vi "Phase_Average_SJ_AM.vi"() -> (5 "Plug in titles":string[](array[string])=["Synthetic_Jet:Frequency:Hz", "Syntehtic_Jet:Num_of:Bins", "Synthetic_Jet:Alanysis:Channels", "Synthetic_Jet:Data:Cluster", "Synethic_Jet:PA_Max_U:U", "Synethic_Jet:PA_Mean_U:U", "Synethic_Jet:PA_Data_Points_Max:U", "Synethic_Jet:PA_Data_Points_Min:U", "Synethic_Jet:PA_Uo:U", "Synethic_Jet:PA_Tb/T:U", "Synethic_Jet:PA_Max_U:V", "Synethic_Jet:PA_Mean_U:V", "Synethic_Jet:PA_Data_Points_Max:V", "Synethic_Jet:PA_Data_Points_Min:V", "Synethic_Jet:PA_Uo:V", "Synethic_Jet:PA_Tb/T:V", "Synethic_Jet:PA_Max_U:Vin", "Synethic_Jet:PA_Mean_U:Vin", "Synethic_Jet:PA_Data_Points_Max:Vin", "Synethic_Jet:PA_Data_Points_Min:Vin", "Synethic_Jet:PA_Max_U:Current", "Synethic_Jet:PA_Mean_U:Current", "Synethic_Jet:PA_Data_Points_Max:Current", "Synethic_Jet:PA_Data_Points_Min:Current", "Synethic_Jet:PA_Max_U:Pressure", "Synethic_Jet:PA_Mean_U:Pressure", "Synethic_Jet:PA_Data_Points_Max:Pressure", "Synethic_Jet:PA_Data_Points_Min:Pressure", "Synethic_Jet:PA_Max_U:Displacement", "Synethic_Jet:PA_Mean_U:Displacement", "Synethic_Jet:PA_Data_Points_Max:Displacement", "Synethic_Jet:PA_Data_Points_Min:Displacement", "Synthetic_Jet:PA_Corr_Coeff:U_cross_V", "Synthetic_Jet:PA_Corr_Coeff_Max:U_cross_V", "Synthetic_Jet:Phase_Lag:U_cross_V", "Synthetic_Jet:PA_Corr_Coeff:U_cross_Vin", "Synthetic_Jet:PA_Corr_Coeff_Max:U_cross_Vin", "Synthetic_Jet:Phase_Lag:U_cross_Vin", "Synthetic_Jet:PA_Corr_Coeff:U_cross_Current", "Synthetic_Jet:PA_Corr_Coeff_Max:U_cross_Current", "Synthetic_Jet:Phase_Lag:U_cross_Current", "Synthetic_Jet:PA_Corr_Coeff:U_cross_Pressure", "Synthetic_Jet:PA_Corr_Coeff_Max:U_cross_Pressure", "Synthetic_Jet:Phase_Lag:U_cross_Pressure", "Synthetic_Jet:PA_Corr_Coeff:U_cross_Displacement", "Synthetic_Jet:PA_Corr_Coeff_Max:U_cross_Displacement", "Synthetic_Jet:Phase_Lag:U_cross_Displacement", "Synthetic_Jet:PA_Corr_Coeff:V_cross_Vin", "Synthetic_Jet:PA_Corr_Coeff_Max:V_cross_Vin", "Synthetic_Jet:Phase_Lag:V_cross_Vin", "Synthetic_Jet:PA_Corr_Coeff:V_cross_Current", "Synthetic_Jet:PA_Corr_Coeff_Max:V_cross_Current", "Synthetic_Jet:Phase_Lag:V_cross_Current", "Synthetic_Jet:PA_Corr_Coeff:V_cross_Pressure", "Synthetic_Jet:PA_Corr_Coeff_Max:V_cross_Pressure", "Synthetic_Jet:Phase_Lag:V_cross_Pressure", "Synthetic_Jet:PA_Corr_Coeff:V_cross_Displacement", "Synthetic_Jet:PA_Corr_Coeff_Max:V_cross_Displacement", "Synthetic_Jet:Phase_Lag:V_cross_Displacement", "Synthetic_Jet:PA_Corr_Coeff:Vin_cross_Current", "Synthetic_Jet:PA_Corr_Coeff_Max:Vin_cross_Current", "Synthetic_Jet:Phase_Lag:Vin_cross_Current", "Synthetic_Jet:PA_Corr_Coeff:Vin_cross_Pressure", "Synthetic_Jet:PA_Corr_Coeff_Max:Vin_cross_Pressure", "Synthetic_Jet:Phase_Lag:Vin_cross_Pressure", "Synthetic_Jet:PA_Corr_Coeff:Vin_cross_Displacement", "Synthetic_Jet:PA_Corr_Coeff_Max:Vin_cross_Displacement", "Synthetic_Jet:Phase_Lag:Vin_cross_Displacement", "Synthetic_Jet:PA_Corr_Coeff:Current_cross_Pressure", "Synthetic_Jet:PA_Corr_Coeff_Max:Current_cross_Pressure", "Synthetic_Jet:Phase_Lag:Current_cross_Pressure", "Synthetic_Jet:PA_Corr_Coeff:Current_cross_Displacement", "Synthetic_Jet:PA_Corr_Coeff_Max:Current_cross_Displacement", "Synthetic_Jet:Phase_Lag:Current_cross_Displacement", "Synthetic_Jet:PA_Corr_Coeff:Pressure_cross_Displacement", "Synthetic_Jet:PA_Corr_Coeff_Max:Pressure_cross_Displacement", "Synthetic_Jet:Phase_Lag:Pressure_cross_Displacement"], 7 "Plug in values":string[](array[string]))   [LabVIEW 2013]
uses:
  Controls/SJ_Data_Cluster.ctl
  Controls/Stats_Menu.ctl
  Controls/Bin_Cluster.ctl
  <vilib>/Analysis/baseanly.llb/Mean (DBL).vi
  <vilib>/Analysis/baseanly.llb/Scale 1D.vi
  <vilib>/Analysis/1siggen.llb/Ramp Pattern by Samples.vi
  Globals/Meas_global.vi
  Globals/Synthetic_jet_global.vi
  <vilib>/Analysis/1siggen.llb/Ramp Pattern by Delta.vi
  <vilib>/Utility/file.llb/Write To Spreadsheet File (DBL).vi
  <vilib>/Analysis/2dsp.llb/1D Cross Correlation (DBL).vi
  <vilib>/Analysis/NI_AALBase.lvlib
  <vilib>/Analysis/NI_AALPro.lvlib
  <vilib>/Analysis/NI_AAL_SigProc.lvlib
panel:
  in  "AM phase Hz":i32=60
  out "Current Frequency":dbl=800.0
  in  "AM Phase averaging?":bool
  in  "Write out PA data?":bool=TRUE
  in  "Tab Control":T1(tab)=enum."Selected Data"
  in  "Overide Channels?":bool
  in  "SJ Data":T2={"Do (mm)"=3.0, "Dc (mm)"=0.039, "Ho (mm)"=0.01, "Hc (mm)"=0.006, "K"=1.251, "beta"=1.039, "Vc (m^3)"=0.0, "Vo (m^3)"=0.0}
  out "Bin Width":dbl=9.693877554482508e-06
  out "Min Num Data Points":i32=548
  in  "Num Bins":i32=20
  in  "Selected Channels":i32[](array[numeric])
  in  "Overide Bins?":bool
  in  "Overide SJ Data":bool
  out "Samples Per Bin":cluster{dbl[], i32[]}[](graph)=[{[0.0, 3.6, 7.2, 10.799999999999999, 14.4, 18.0, 21.599999999999998, 25.200000000000003, 28.8, 32.4, 36.0, 39.6, 43.199999999999996, 46.800000000000004, 50.400000000000006, 54.0, 57.6, 61.2, 64.8, 68.4, 72.0, 75.6, 79.2, 82.8, 86.39999999999999, 90.0, 93.60000000000001, 97.2, 100.80000000000001, 104.39999999999999, 108.0, 111.6, 115.2, 118.80000000000001, 122.4, 126.00000000000001, 129.6, 133.2, 136.8, 140.4, 144.0, 147.60000000000002, 151.2, 154.8, 158.4, 162.0, 165.6, 169.20000000000002, 172.79999999999998, 176.4, 180.0, 183.6, 187.20000000000002, 190.8, 194.4, 198.00000000000003, 201.60000000000002, 205.20000000000002, 208.79999999999998, 212.39999999999998, 216.0, 219.6, 223.2, 226.8, 230.4, 234.0, 237.60000000000002, 241.20000000000002, 244.8, 248.40000000000003, 252.00000000000003, 255.6, 259.2, 262.8, 266.4, 270.0, 273.6, 277.2, 280.8, 284.40000000000003, 288.0, 291.6, 295.20000000000005, 298.8, 302.4, 306.0, 309.6, 313.2, 316.8, 320.4, 324.0, 327.6, 331.2, 334.8, 338.40000000000003, 342.0, 345.59999999999997, 349.2, 352.8, 356.4], [1358, 1345, 1296, 1279, 1181, 1241, 1218, 1082, 1071, 960, 945, 848, 827, 742, 747, 751, 677, 739, 745, 766, 766, 737, 764, 790, 872, 945, 1003, 1066, 1169, 1174, 1250, 1309, 1280, 1388, 1423, 1525, 1537, 1567, 1651, 1571, 1663, 1750, 1677, 1743, 1772, 1705, 1797, 1760, 1746, 1725, 1725, 1747, 1685, 1690, 1563, 1571, 1574, 1487, 1458, 1301, 1305, 1275, 1247, 1196, 1110, 1139, 1029, 969, 995, 960, 948, 839, 925, 938, 862, 860, 943, 895, 990, 971, 984, 1037, 1058, 1109, 1122, 1164, 1278, 1226, 1300, 1339, 1395, 1341, 1435, 1376, 1395, 1372, 1444, 1337, 1357, 1373]}, {[0.0, 3.6, 7.2, 10.799999999999999, 14.4, 18.0, 21.599999999999998, 25.200000000000003, 28.8, 32.4, 36.0, 39.6, 43.199999999999996, 46.800000000000004, 50.400000000000006, 54.0, 57.6, 61.2, 64.8, 68.4, 72.0, 75.6, 79.2, 82.8, 86.39999999999999, 90.0, 93.60000000000001, 97.2, 100.80000000000001, 104.39999999999999, 108.0, 111.6, 115.2, 118.80000000000001, 122.4, 126.00000000000001, 129.6, 133.2, 136.8, 140.4, 144.0, 147.60000000000002, 151.2, 154.8, 158.4, 162.0, 165.6, 169.20000000000002, 172.79999999999998, 176.4, 180.0, 183.6, 187.20000000000002, 190.8, 194.4, 198.00000000000003, 201.60000000000002, 205.20000000000002, 208.79999999999998, 212.39999999999998, 216.0, 219.6, 223.2, 226.8, 230.4, 234.0, 237.60000000000002, 241.20000000000002, 244.8, 248.40000000000003, 252.00000000000003, 255.6, 259.2, 262.8, 266.4, 270.0, 273.6, 277.2, 280.8, 284.40000000000003, 288.0, 291.6, 295.20000000000005, 298.8, 302.4, 306.0, 309.6, 313.2, 316.8, 320.4, 324.0, 327.6, 331.2, 334.8, 338.40000000000003, 342.0, 345.59999999999997, 349.2, 352.8, 356.4], [1147, 1108, 1116, 1075, 1046, 958, 984, 885, 882, 753, 768, 693, 636, 559, 548, 565, 563, 574, 560, 596, 594, 638, 613, 636, 694, 743, 822, 895, 958, 1079, 1079, 1156, 1163, 1207, 1247, 1248, 1289, 1304, 1365, 1443, 1428, 1457, 1436, 1501, 1564, 1476, 1494, 1421, 1495, 1460, 1460, 1447, 1439, 1424, 1392, 1304, 1278, 1228, 1237, 1132, 1047, 985, 968, 932, 908, 819, 819, 753, 702, 627, 641, 648, 609, 630, 643, 665, 682, 724, 722, 764, 788, 784, 821, 842, 888, 918, 937, 1005, 1043, 1079, 1132, 1099, 1179, 1079, 1153, 1158, 1160, 1177, 1142, 1156]}, {[0.0, 3.6, 7.2, 10.799999999999999, 14.4, 18.0, 21.599999999999998, 25.200000000000003, 28.8, 32.4, 36.0, 39.6, 43.199999999999996, 46.800000000000004, 50.400000000000006, 54.0, 57.6, 61.2, 64.8, 68.4, 72.0, 75.6, 79.2, 82.8, 86.39999999999999, 90.0, 93.60000000000001, 97.2, 100.80000000000001, 104.39999999999999, 108.0, 111.6, 115.2, 118.80000000000001, 122.4, 126.00000000000001, 129.6, 133.2, 136.8, 140.4, 144.0, 147.60000000000002, 151.2, 154.8, 158.4, 162.0, 165.6, 169.20000000000002, 172.79999999999998, 176.4, 180.0, 183.6, 187.20000000000002, 190.8, 194.4, 198.00000000000003, 201.60000000000002, 205.20000000000002, 208.79999999999998, 212.39999999999998, 216.0, 219.6, 223.2, 226.8, 230.4, 234.0, 237.60000000000002, 241.20000000000002, 244.8, 248.40000000000003, 252.00000000000003, 255.6, 259.2, 262.8, 266.4, 270.0, 273.6, 277.2, 280.8, 284.40000000000003, 288.0, 291.6, 295.20000000000005, 298.8, 302.4, 306.0, 309.6, 313.2, 316.8, 320.4, 324.0, 327.6, 331.2, 334.8, 338.40000000000003, 342.0, 345.59999999999997, 349.2, 352.8, 356.4], [1604, 1604, 1600, 1600, 1600, 1608, 1600, 1600, 1600, 1604, 1604, 1604, 1596, 1604, 1600, 1600, 1604, 1600, 1600, 1600, 1604, 1600, 1600, 1604, 1596, 1604, 1604, 1600, 1600, 1600, 1596, 1604, 1592, 1596, 1608, 1600, 1600, 1604, 1596, 1604, 1604, 1600, 1596, 1604, 1604, 1600, 1600, 1600, 1600, 1608, 1596, 1600, 1604, 1600, 1604, 1600, 1596, 1604, 1604, 1600, 1596, 1604, 1600, 1600, 1600, 1596, 1596, 1604, 1600, 1604, 1600, 1596, 1604, 1604, 1600, 1604, 1596, 1600, 1608, 1600, 1596, 1600, 1604, 1604, 1600, 1600, 1596, 1608, 1604, 1596, 1600, 1600, 1604, 1608, 1592, 1600, 1604, 1596, 1596, 1600]}, {[0.0, 3.6, 7.2, 10.799999999999999, 14.4, 18.0, 21.599999999999998, 25.200000000000003, 28.8, 32.4, 36.0, 39.6, 43.199999999999996, 46.800000000000004, 50.400000000000006, 54.0, 57.6, 61.2, 64.8, 68.4, 72.0, 75.6, 79.2, 82.8, 86.39999999999999, 90.0, 93.60000000000001, 97.2, 100.80000000000001, 104.39999999999999, 108.0, 111.6, 115.2, 118.80000000000001, 122.4, 126.00000000000001, 129.6, 133.2, 136.8, 140.4, 144.0, 147.60000000000002, 151.2, 154.8, 158.4, 162.0, 165.6, 169.20000000000002, 172.79999999999998, 176.4, 180.0, 183.6, 187.20000000000002, 190.8, 194.4, 198.00000000000003, 201.60000000000002, 205.20000000000002, 208.79999999999998, 212.39999999999998, 216.0, 219.6, 223.2, 226.8, 230.4, 234.0, 237.60000000000002, 241.20000000000002, 244.8, 248.40000000000003, 252.00000000000003, 255.6, 259.2, 262.8, 266.4, 270.0, 273.6, 277.2, 280.8, 284.40000000000003, 288.0, 291.6, 295.20000000000005, 298.8, 302.4, 306.0, 309.6, 313.2, 316.8, 320.4, 324.0, 327.6, 331.2, 334.8, 338.40000000000003, 342.0, 345.59999999999997, 349.2, 352.8, 356.4], [1604, 1604, 1600, 1600, 1600, 1608, 1600, 1600, 1600, 1604, 1604, 1604, 1596, 1604, 1600, 1600, 1604, 1600, 1600, 1600, 1604, 1600, 1600, 1604, 1596, 1604, 1604, 1600, 1600, 1600, 1596, 1604, 1592, 1596, 1608, 1600, 1600, 1604, 1596, 1604, 1604, 1600, 1596, 1604, 1604, 1600, 1600, 1600, 1600, 1608, 1596, 1600, 1604, 1600, 1604, 1600, 1596, 1604, 1604, 1600, 1596, 1604, 1600, 1600, 1600, 1596, 1596, 1604, 1600, 1604, 1600, 1596, 1604, 1604, 1600, 1604, 1596, 1600, 1608, 1600, 1596, 1600, 1604, 1604, 1600, 1600, 1596, 1608, 1604, 1596, 1600, 1600, 1604, 1608, 1592, 1600, 1604, 1596, 1596, 1600]}, {[0.0, 3.6, 7.2, 10.799999999999999, 14.4, 18.0, 21.599999999999998, 25.200000000000003, 28.8, 32.4, 36.0, 39.6, 43.199999999999996, 46.800000000000004, 50.400000000000006, 54.0, 57.6, 61.2, 64.8, 68.4, 72.0, 75.6, 79.2, 82.8, 86.39999999999999, 90.0, 93.60000000000001, 97.2, 100.80000000000001, 104.39999999999999, 108.0, 111.6, 115.2, 118.80000000000001, 122.4, 126.00000000000001, 129.6, 133.2, 136.8, 140.4, 144.0, 147.60000000000002, 151.2, 154.8, 158.4, 162.0, 165.6, 169.20000000000002, 172.79999999999998, 176.4, 180.0, 183.6, 187.20000000000002, 190.8, 194.4, 198.00000000000003, 201.60000000000002, 205.20000000000002, 208.79999999999998, 212.39999999999998, 216.0, 219.6, 223.2, 226.8, 230.4, 234.0, 237.60000000000002, 241.20000000000002, 244.8, 248.40000000000003, 252.00000000000003, 255.6, 259.2, 262.8, 266.4, 270.0, 273.6, 277.2, 280.8, 284.40000000000003, 288.0, 291.6, 295.20000000000005, 298.8, 302.4, 306.0, 309.6, 313.2, 316.8, 320.4, 324.0, 327.6, 331.2, 334.8, 338.40000000000003, 342.0, 345.59999999999997, 349.2, 352.8, 356.4], [1604, 1604, 1600, 1600, 1600, 1608, 1600, 1600, 1600, 1604, 1604, 1604, 1596, 1604, 1600, 1600, 1604, 1600, 1600, 1600, 1604, 1600, 1600, 1604, 1596, 1604, 1604, 1600, 1600, 1600, 1596, 1604, 1592, 1596, 1608, 1600, 1600, 1604, 1596, 1604, 1604, 1600, 1596, 1604, 1604, 1600, 1600, 1600, 1600, 1608, 1596, 1600, 1604, 1600, 1604, 1600, 1596, 1604, 1604, 1600, 1596, 1604, 1600, 1600, 1600, 1596, 1596, 1604, 1600, 1604, 1600, 1596, 1604, 1604, 1600, 1604, 1596, 1600, 1608, 1600, 1596, 1600, 1604, 1604, 1600, 1600, 1596, 1608, 1604, 1596, 1600, 1600, 1604, 1608, 1592, 1600, 1604, 1596, 1596, 1600]}, {[0.0, 3.6, 7.2, 10.799999999999999, 14.4, 18.0, 21.599999999999998, 25.200000000000003, 28.8, 32.4, 36.0, 39.6, 43.199999999999996, 46.800000000000004, 50.400000000000006, 54.0, 57.6, 61.2, 64.8, 68.4, 72.0, 75.6, 79.2, 82.8, 86.39999999999999, 90.0, 93.60000000000001, 97.2, 100.80000000000001, 104.39999999999999, 108.0, 111.6, 115.2, 118.80000000000001, 122.4, 126.00000000000001, 129.6, 133.2, 136.8, 140.4, 144.0, 147.60000000000002, 151.2, 154.8, 158.4, 162.0, 165.6, 169.20000000000002, 172.79999999999998, 176.4, 180.0, 183.6, 187.20000000000002, 190.8, 194.4, 198.00000000000003, 201.60000000000002, 205.20000000000002, 208.79999999999998, 212.39999999999998, 216.0, 219.6, 223.2, 226.8, 230.4, 234.0, 237.60000000000002, 241.20000000000002, 244.8, 248.40000000000003, 252.00000000000003, 255.6, 259.2, 262.8, 266.4, 270.0, 273.6, 277.2, 280.8, 284.40000000000003, 288.0, 291.6, 295.20000000000005, 298.8, 302.4, 306.0, 309.6, 313.2, 316.8, 320.4, 324.0, 327.6, 331.2, 334.8, 338.40000000000003, 342.0, 345.59999999999997, 349.2, 352.8, 356.4], [1604, 1604, 1600, 1600, 1600, 1608, 1600, 1600, 1600, 1604, 1604, 1604, 1596, 1604, 1600, 1600, 1604, 1600, 1600, 1600, 1604, 1600, 1600, 1604, 1596, 1604, 1604, 1600, 1600, 1600, 1596, 1604, 1592, 1596, 1608, 1600, 1600, 1604, 1596, 1604, 1604, 1600, 1596, 1604, 1604, 1600, 1600, 1600, 1600, 1608, 1596, 1600, 1604, 1600, 1604, 1600, 1596, 1604, 1604, 1600, 1596, 1604, 1600, 1600, 1600, 1596, 1596, 1604, 1600, 1604, 1600, 1596, 1604, 1604, 1600, 1604, 1596, 1600, 1608, 1600, 1596, 1600, 1604, 1604, 1600, 1600, 1596, 1608, 1604, 1596, 1600, 1600, 1604, 1608, 1592, 1600, 1604, 1596, 1596, 1600]}]
  out "Engineering Values Scaled":cluster{dbl[], "Y=(X-offset)/scale":dbl[]}[](graph)=[{[0.0, 3.6, 7.2, 10.799999999999999, 14.4, 18.0, 21.599999999999998, 25.200000000000003, 28.8, 32.4, 36.0, 39.6, 43.199999999999996, 46.800000000000004, 50.400000000000006, 54.0, 57.6, 61.2, 64.8, 68.4, 72.0, 75.6, 79.2, 82.8, 86.39999999999999, 90.0, 93.60000000000001, 97.2, 100.80000000000001, 104.39999999999999, 108.0, 111.6, 115.2, 118.80000000000001, 122.4, 126.00000000000001, 129.6, 133.2, 136.8, 140.4, 144.0, 147.60000000000002, 151.2, 154.8, 158.4, 162.0, 165.6, 169.20000000000002, 172.79999999999998, 176.4, 180.0, 183.6, 187.20000000000002, 190.8, 194.4, 198.00000000000003, 201.60000000000002, 205.20000000000002, 208.79999999999998, 212.39999999999998, 216.0, 219.6, 223.2, 226.8, 230.4, 234.0, 237.60000000000002, 241.20000000000002, 244.8, 248.40000000000003, 252.00000000000003, 255.6, 259.2, 262.8, 266.4, 270.0, 273.6, 277.2, 280.8, 284.40000000000003, 288.0, 291.6, 295.20000000000005, 298.8, 302.4, 306.0, 309.6, 313.2, 316.8, 320.4, 324.0, 327.6, 331.2, 334.8, 338.40000000000003, 342.0, 345.59999999999997, 349.2, 352.8, 356.4], "Y=(X-offset)/scale"=[-0.9551153818154593, -0.9386708768164268, -0.9149482127660302, -0.8827086653672397, -0.8571546888473836, -0.8212304216223307, -0.7845060998363727, -0.748651473112596, -0.7025889549208455, -0.6484101862421825, -0.6020642757553747, -0.5570629113828607, -0.48394929325128827, -0.4161715285035951, -0.35985820573777677, -0.2971562326810696, -0.23383278861290493, -0.1878049478017613, -0.14399418919574525, -0.10176114549965982, -0.05340825159098972, 0.0031119310172862944, 0.0898140329754603, 0.16655011360172153, 0.2335979115701082, 0.2849005543486347, 0.3395231481920418, 0.37670823157269784, 0.43078592238789737, 0.4894409536702755, 0.5308781549353541, 0.5685469269508053, 0.6121523593369985, 0.6549610151521917, 0.6906786996134701, 0.7304874396585026, 0.7772210570077172, 0.7921324647883226, 0.8357876373822483, 0.8726159685492605, 0.8971448098950745, 0.9112423741948901, 0.9387797319740145, 0.9692072065965601, 0.9806209311434405, 0.9802782784752133, 0.982207601694826, 1.0, 0.9923989104538731, 0.9934869697759626, 0.99168135356283, 0.9699166080066824, 0.9465766839373022, 0.9361942960185334, 0.8614870493369937, 0.841171792656405, 0.8129017211569531, 0.7586134580175187, 0.7066499984875707, 0.6716334546351881, 0.60763394011458, 0.538615622218619, 0.46465943995624104, 0.43650233431712127, 0.33454310017245303, 0.3037987239608861, 0.21848497259253033, 0.13518581261223045, 0.10287130243872596, 0.035598747439908165, -0.0422264980405214, -0.11750774774481676, -0.1632930691402038, -0.23950339955887318, -0.2858830534794818, -0.36181374962243146, -0.38659174412235037, -0.42025876301264853, -0.49695360086112367, -0.5489646663866689, -0.5999064227716845, -0.66043042114079, -0.7012963181146216, -0.7535927425911034, -0.7947263878889465, -0.8028301348596579, -0.852104364406295, -0.8696631708281138, -0.8996700970639971, -0.935762520845454, -0.9496371590192277, -0.9516459155006031, -0.9763778733099013, -0.9792522871844971, -0.9968488820233004, -1.0, -0.982250992744951, -0.9920432258770852, -0.9810909213509464, -0.9782577963358422]}, {[0.0, 3.6, 7.2, 10.799999999999999, 14.4, 18.0, 21.599999999999998, 25.200000000000003, 28.8, 32.4, 36.0, 39.6, 43.199999999999996, 46.800000000000004, 50.400000000000006, 54.0, 57.6, 61.2, 64.8, 68.4, 72.0, 75.6, 79.2, 82.8, 86.39999999999999, 90.0, 93.60000000000001, 97.2, 100.80000000000001, 104.39999999999999, 108.0, 111.6, 115.2, 118.80000000000001, 122.4, 126.00000000000001, 129.6, 133.2, 136.8, 140.4, 144.0, 147.60000000000002, 151.2, 154.8, 158.4, 162.0, 165.6, 169.20000000000002, 172.79999999999998, 176.4, 180.0, 183.6, 187.20000000000002, 190.8, 194.4, 198.00000000000003, 201.60000000000002, 205.20000000000002, 208.79999999999998, 212.39999999999998, 216.0, 219.6, 223.2, 226.8, 230.4, 234.0, 237.60000000000002, 241.20000000000002, 244.8, 248.40000000000003, 252.00000000000003, 255.6, 259.2, 262.8, 266.4, 270.0, 273.6, 277.2, 280.8, 284.40000000000003, 288.0, 291.6, 295.20000000000005, 298.8, 302.4, 306.0, 309.6, 313.2, 316.8, 320.4, 324.0, 327.6, 331.2, 334.8, 338.40000000000003, 342.0, 345.59999999999997, 349.2, 352.8, 356.4], "Y=(X-offset)/scale"=[-0.6000257655960964, -0.6296084547831131, -0.5644188522659417, -0.5471668426469449, -0.5301005517796318, -0.5217383066292558, -0.4622577642837686, -0.3879637776401403, -0.41150371567583416, -0.3919780554602071, -0.34346035985346257, -0.254251186050764, -0.16933160610108522, -0.16358783981514913, -0.19775129670736702, -0.11171513893076099, -0.07987388867123553, -0.0038315286054692336, -0.04427218846366556, 0.04326943351900303, 0.06364948012281159, 0.04439754383546602, 0.13634659123892143, 0.2018024685577136, 0.28603171816787276, 0.25359032504604373, 0.30261797802126983, 0.37211497845990044, 0.38811857241522246, 0.47416342564524555, 0.48855942251936385, 0.509681101698175, 0.548928600269913, 0.5762077937057899, 0.623049168889291, 0.65962227137938, 0.7496236779793469, 0.6835564674541392, 0.7872377845809949, 0.8752846647101659, 0.9058482192741587, 0.9024524092422583, 0.9954677709139663, 0.8961181525300512, 1.0, 0.9126293702045721, 0.9513759030893776, 0.9082778122911612, 0.8899531986178352, 0.8542600336388043, 0.8869169285396474, 0.7872321008706873, 0.7618678948362775, 0.6769274050542455, 0.5582685539747775, 0.5318027924828322, 0.3768582075706238, 0.3905102299559355, 0.246521072626692, 0.23616866065979547, 0.10754072961511849, 0.07637840202411009, -0.009571846812151478, -0.16938387752406225, -0.08186540292904956, -0.2733266546034608, -0.3631519879569536, -0.3332127098152006, -0.4563965670684298, -0.5602929817749812, -0.432730610080142, -0.5873973221989619, -0.6776048246187775, -0.6842771834265521, -0.6171245381295548, -0.751123919185737, -0.6775780134848866, -0.6411087785539201, -0.8185144122575803, -0.8082595763243787, -0.8601856909719153, -0.9281689486568823, -0.9399487973293656, -0.9558082481365745, -0.9361486165062145, -0.9404541937899846, -1.0, -0.9254977324397713, -0.9007846729344119, -0.9319768254925832, -0.8836209796140401, -0.8008104857946138, -0.9022650900561288, -0.7892983407156048, -0.802189877344158, -0.7374909344930695, -0.7165791211179161, -0.666500904887512, -0.6822185692774972, -0.737008511025971]}, {[0.0, 3.6, 7.2, 10.799999999999999, 14.4, 18.0, 21.599999999999998, 25.200000000000003, 28.8, 32.4, 36.0, 39.6, 43.199999999999996, 46.800000000000004, 50.400000000000006, 54.0, 57.6, 61.2, 64.8, 68.4, 72.0, 75.6, 79.2, 82.8, 86.39999999999999, 90.0, 93.60000000000001, 97.2, 100.80000000000001, 104.39999999999999, 108.0, 111.6, 115.2, 118.80000000000001, 122.4, 126.00000000000001, 129.6, 133.2, 136.8, 140.4, 144.0, 147.60000000000002, 151.2, 154.8, 158.4, 162.0, 165.6, 169.20000000000002, 172.79999999999998, 176.4, 180.0, 183.6, 187.20000000000002, 190.8, 194.4, 198.00000000000003, 201.60000000000002, 205.20000000000002, 208.79999999999998, 212.39999999999998, 216.0, 219.6, 223.2, 226.8, 230.4, 234.0, 237.60000000000002, 241.20000000000002, 244.8, 248.40000000000003, 252.00000000000003, 255.6, 259.2, 262.8, 266.4, 270.0, 273.6, 277.2, 280.8, 284.40000000000003, 288.0, 291.6, 295.20000000000005, 298.8, 302.4, 306.0, 309.6, 313.2, 316.8, 320.4, 324.0, 327.6, 331.2, 334.8, 338.40000000000003, 342.0, 345.59999999999997, 349.2, 352.8, 356.4], "Y=(X-offset)/scale"=[-0.324332635145967, -0.3838198713757219, -0.44081635783682965, -0.49677620053035504, -0.5506176190745422, -0.6016412934008409, -0.6510998236349615, -0.6979186329701068, -0.7408503368561451, -0.7823676502632549, -0.8194289332341465, -0.8538505515393717, -0.8852000566796311, -0.9121357432391195, -0.9365447196039366, -0.9563984945596902, -0.9730569223136102, -0.9855999607686946, -0.9940970958857072, -0.9990580460582431, -1.0, -0.9969372982284642, -0.9900730345704503, -0.9790274583582089, -0.9647344799818981, -0.9460722420888912, -0.9238348078458232, -0.8981293358072846, -0.8685193839184734, -0.8362910192677246, -0.8004211709195546, -0.7610585566664713, -0.7188260754084056, -0.6742369082784718, -0.6265183604012093, -0.5760227440012722, -0.5243522754029674, -0.46856698484684417, -0.4116453200341878, -0.35429697815097067, -0.29438956022332385, -0.23404576059030877, -0.17156181549709187, -0.10965470570481395, -0.046520785865849255, 0.016289322156093303, 0.0782112916621511, 0.14265292590520148, 0.20374035832669787, 0.2652043243472213, 0.32496108551551306, 0.38355755257856, 0.4416600727262193, 0.4970807895566517, 0.5502506998787882, 0.6011085558610448, 0.6503974820545738, 0.6966019309972807, 0.7404334683585393, 0.7809450544956844, 0.8184384115998369, 0.8528818222435408, 0.8838389751352131, 0.9116270989672535, 0.935110787289453, 0.9559393293824295, 0.9720488882455951, 0.9846819898204856, 0.9939115813890408, 0.9989718552474046, 1.0, 0.9974545776418189, 0.9905248186412435, 0.9797572518002684, 0.9653321284070773, 0.9469355392532751, 0.9247748338013451, 0.8990806357040502, 0.8694072459887088, 0.8364925462174618, 0.8007713907470402, 0.7612211647205798, 0.719129817142212, 0.6734979383918018, 0.6256834923978529, 0.5751178905260256, 0.5226125738268346, 0.4681770170126485, 0.41060550382546346, 0.35334796890568226, 0.29262025753632986, 0.23285060362745555, 0.1712713479675681, 0.10787688697628549, 0.04551789324166519, -0.017619594059556206, -0.07995233700932476, -0.14130155409470893, -0.20370375735350435, -0.26591530181050727]}, {[0.0, 3.6, 7.2, 10.799999999999999, 14.4, 18.0, 21.599999999999998, 25.200000000000003, 28.8, 32.4, 36.0, 39.6, 43.199999999999996, 46.800000000000004, 50.400000000000006, 54.0, 57.6, 61.2, 64.8, 68.4, 72.0, 75.6, 79.2, 82.8, 86.39999999999999, 90.0, 93.60000000000001, 97.2, 100.80000000000001, 104.39999999999999, 108.0, 111.6, 115.2, 118.80000000000001, 122.4, 126.00000000000001, 129.6, 133.2, 136.8, 140.4, 144.0, 147.60000000000002, 151.2, 154.8, 158.4, 162.0, 165.6, 169.20000000000002, 172.79999999999998, 176.4, 180.0, 183.6, 187.20000000000002, 190.8, 194.4, 198.00000000000003, 201.60000000000002, 205.20000000000002, 208.79999999999998, 212.39999999999998, 216.0, 219.6, 223.2, 226.8, 230.4, 234.0, 237.60000000000002, 241.20000000000002, 244.8, 248.40000000000003, 252.00000000000003, 255.6, 259.2, 262.8, 266.4, 270.0, 273.6, 277.2, 280.8, 284.40000000000003, 288.0, 291.6, 295.20000000000005, 298.8, 302.4, 306.0, 309.6, 313.2, 316.8, 320.4, 324.0, 327.6, 331.2, 334.8, 338.40000000000003, 342.0, 345.59999999999997, 349.2, 352.8, 356.4], "Y=(X-offset)/scale"=[-0.999477163867277, -1.0, -0.995833837226098, -0.987898747711675, -0.9753734782715575, -0.9591109182029777, -0.938151115815857, -0.9125929181274602, -0.8834560187312184, -0.8489540333199225, -0.8113916998804199, -0.7695338948729418, -0.7240212666116366, -0.6751376300648789, -0.6223626043144008, -0.5680576186970898, -0.5093095314549057, -0.45057763189459554, -0.38870492872574386, -0.325563456299371, -0.2619475442118494, -0.1959196004083376, -0.1315246843879441, -0.06550485068778504, -0.0021499839154213974, 0.06250834085357543, 0.12457836354506895, 0.18593497538706555, 0.2468153361851179, 0.304587456519989, 0.3615037199868826, 0.41776563104806347, 0.47191895369797676, 0.525011810821948, 0.5755782254341417, 0.6254791331531085, 0.6726956683858427, 0.7191932235530573, 0.7624612688694594, 0.8024041654586451, 0.8400249951807948, 0.8739991890717225, 0.9049408992943399, 0.9313591827122311, 0.9536605117952182, 0.9722781758441066, 0.9860929682515216, 0.9955044678806833, 1.0, 0.9993700137544395, 0.994782094536492, 0.9845809980139224, 0.9697232160151795, 0.9504828474978425, 0.9267307827026403, 0.8993530995614197, 0.8669074775421599, 0.8310851243856565, 0.7918109498119879, 0.7488005048544422, 0.703120115856144, 0.6538080238541689, 0.6025128602542822, 0.5484536263860987, 0.49356912784581364, 0.434318748401323, 0.37703129357358267, 0.31744177168835014, 0.25639689829473994, 0.19636228737389466, 0.13565546010338472, 0.07654853738280328, 0.016945513710682387, -0.04101262290395395, -0.09721489387748518, -0.15191465245710603, -0.2062248937225819, -0.25742165674798384, -0.3079563420450002, -0.35705295347058436, -0.40376923853247726, -0.4498426508681331, -0.4943670108445233, -0.5385492834293556, -0.5806889870930813, -0.6226507252858628, -0.6625263962192042, -0.7011898025065944, -0.7389349961378829, -0.7742398969292655, -0.8091261898864373, -0.8399709398002756, -0.8691024946886746, -0.8967180235917159, -0.9214150454408416, -0.9430295872576268, -0.9607977861913224, -0.9758975154254286, -0.9872712381476475, -0.995898000505844]}, {[0.0, 3.6, 7.2, 10.799999999999999, 14.4, 18.0, 21.599999999999998, 25.200000000000003, 28.8, 32.4, 36.0, 39.6, 43.199999999999996, 46.800000000000004, 50.400000000000006, 54.0, 57.6, 61.2, 64.8, 68.4, 72.0, 75.6, 79.2, 82.8, 86.39999999999999, 90.0, 93.60000000000001, 97.2, 100.80000000000001, 104.39999999999999, 108.0, 111.6, 115.2, 118.80000000000001, 122.4, 126.00000000000001, 129.6, 133.2, 136.8, 140.4, 144.0, 147.60000000000002, 151.2, 154.8, 158.4, 162.0, 165.6, 169.20000000000002, 172.79999999999998, 176.4, 180.0, 183.6, 187.20000000000002, 190.8, 194.4, 198.00000000000003, 201.60000000000002, 205.20000000000002, 208.79999999999998, 212.39999999999998, 216.0, 219.6, 223.2, 226.8, 230.4, 234.0, 237.60000000000002, 241.20000000000002, 244.8, 248.40000000000003, 252.00000000000003, 255.6, 259.2, 262.8, 266.4, 270.0, 273.6, 277.2, 280.8, 284.40000000000003, 288.0, 291.6, 295.20000000000005, 298.8, 302.4, 306.0, 309.6, 313.2, 316.8, 320.4, 324.0, 327.6, 331.2, 334.8, 338.40000000000003, 342.0, 345.59999999999997, 349.2, 352.8, 356.4], "Y=(X-offset)/scale"=[0.24798886036906698, 0.30694086077660476, 0.3642095468100585, 0.4212388206223648, 0.4772455735602993, 0.5311088513860781, 0.5843671486103762, 0.6358303072039728, 0.6837980481639937, 0.7310432746524327, 0.7737311958300097, 0.8140957953828596, 0.8510643564392585, 0.882952084279465, 0.9121717576229643, 0.9362761032577382, 0.9566418759813594, 0.9728068048999052, 0.9847297456081049, 0.9932059588740203, 0.9982521215535534, 1.0, 0.9985958788235885, 0.9941830996390469, 0.987120440473217, 0.9769411681055087, 0.9637931320950248, 0.9479205541098594, 0.9286125464455226, 0.9066092471942216, 0.8811045375226862, 0.8515787428062843, 0.8185573409961007, 0.7822134336490338, 0.7416779590856867, 0.6973765058637093, 0.6505950238320156, 0.5985543258925514, 0.5444814356995393, 0.4888205952477875, 0.4298488359060673, 0.3700411729571332, 0.30752228271061893, 0.2453949285457375, 0.18206421313080534, 0.11903705068725319, 0.057139439971723265, -0.007220101030625045, -0.06813067822715113, -0.1295563755840377, -0.18991733891747972, -0.2494230240775392, -0.30955326493446883, -0.3679785421329789, -0.42548046869675754, -0.4820539905587055, -0.5383762168301456, -0.592769088326793, -0.645628167253372, -0.6956777887504435, -0.7430103899338654, -0.7875506147216481, -0.8280771682974074, -0.8650755752817957, -0.8967911032150638, -0.9254198000347772, -0.948212438469826, -0.9669527091292689, -0.9818466144977595, -0.9920200114248434, -0.9977552151391165, -1.0, -0.9981145809461024, -0.9926946393873112, -0.9840652554597449, -0.9717188643000962, -0.9563437929329474, -0.9374004474906461, -0.914585720841493, -0.8887684842397121, -0.8593105672967526, -0.8257209527528148, -0.7887117372658937, -0.7469700250041118, -0.7020904875255574, -0.6529034827799842, -0.6007122397849494, -0.5454247553519498, -0.4861743282108634, -0.4270266091724415, -0.3642359772912829, -0.3024703661156339, -0.23973300672637374, -0.17567688289612113, -0.1134144061952939, -0.05130225676736532, 0.009671750947260563, 0.06933608631330149, 0.12995528015626395, 0.19053569191894756]}, {[0.0, 3.6, 7.2, 10.799999999999999, 14.4, 18.0, 21.599999999999998, 25.200000000000003, 28.8, 32.4, 36.0, 39.6, 43.199999999999996, 46.800000000000004, 50.400000000000006, 54.0, 57.6, 61.2, 64.8, 68.4, 72.0, 75.6, 79.2, 82.8, 86.39999999999999, 90.0, 93.60000000000001, 97.2, 100.80000000000001, 104.39999999999999, 108.0, 111.6, 115.2, 118.80000000000001, 122.4, 126.00000000000001, 129.6, 133.2, 136.8, 140.4, 144.0, 147.60000000000002, 151.2, 154.8, 158.4, 162.0, 165.6, 169.20000000000002, 172.79999999999998, 176.4, 180.0, 183.6, 187.20000000000002, 190.8, 194.4, 198.00000000000003, 201.60000000000002, 205.20000000000002, 208.79999999999998, 212.39999999999998, 216.0, 219.6, 223.2, 226.8, 230.4, 234.0, 237.60000000000002, 241.20000000000002, 244.8, 248.40000000000003, 252.00000000000003, 255.6, 259.2, 262.8, 266.4, 270.0, 273.6, 277.2, 280.8, 284.40000000000003, 288.0, 291.6, 295.20000000000005, 298.8, 302.4, 306.0, 309.6, 313.2, 316.8, 320.4, 324.0, 327.6, 331.2, 334.8, 338.40000000000003, 342.0, 345.59999999999997, 349.2, 352.8, 356.4], "Y=(X-offset)/scale"=[-0.9740279920181284, -0.9846373610513185, -0.993320779441793, -0.9981881422032391, -1.0, -0.9985034423533582, -0.9966436575584205, -0.9948478632283323, -0.9888871672778952, -0.9802074776349564, -0.9708220034750391, -0.9598702874710158, -0.9472496837993849, -0.9318059159059814, -0.9165205641568439, -0.8989799834382035, -0.8787821491656113, -0.8557927595533076, -0.8321828629012147, -0.8071867299816438, -0.778083232433784, -0.7452078131757824, -0.7114712514890126, -0.6727963459650614, -0.6358055098454907, -0.5922837693334781, -0.5472900118366004, -0.49845943357685313, -0.44754200739559946, -0.39850108326512357, -0.34071476098245435, -0.28347567543415353, -0.22251156195994248, -0.16025195206529771, -0.09802186457986746, -0.03155074190368913, 0.032933808330448476, 0.09959109990319813, 0.16678387404418069, 0.23170146358040958, 0.2950335529132527, 0.35845059714725863, 0.4221270154547499, 0.4819989498155311, 0.5381272323377648, 0.5937365353181965, 0.6457901127738864, 0.6974173369464612, 0.7430674916254536, 0.7896290662788872, 0.8300966893376822, 0.8658249474641341, 0.8982686678667795, 0.9279886120282342, 0.9517741984536113, 0.9717513200542929, 0.9852076702205445, 0.9935630444457303, 1.0, 0.9985171650156098, 0.9922135823209215, 0.9835195039994218, 0.9659403209003125, 0.9461292272727337, 0.9200738168538403, 0.8888674276141129, 0.8498067287997931, 0.8117016667430699, 0.7676870036846396, 0.7141748224755682, 0.6604419498718704, 0.6031335003313849, 0.5428168228520944, 0.4771021367227203, 0.4102029794093248, 0.3388377246912229, 0.2678194184920453, 0.1941434987296745, 0.1200453795998981, 0.04349414815145887, -0.029161554569596376, -0.10413288709716835, -0.17498213828263112, -0.24626789528944998, -0.31451590225673404, -0.3824643427235468, -0.44559201683689925, -0.503743365423006, -0.5628367808231299, -0.6163875399650314, -0.6681927885891562, -0.7150617434577229, -0.7594872366097571, -0.8009598502582057, -0.8366271303783458, -0.8694097045479963, -0.8969538126221946, -0.9223926903176659, -0.9404960974508143, -0.961060804521041]}]
  out "Engineering Values":cluster{dbl[], dbl[]}(graph)={[0.0, 3.6, 7.2, 10.799999999999999, 14.4, 18.0, 21.599999999999998, 25.200000000000003, 28.8, 32.4, 36.0, 39.6, 43.199999999999996, 46.800000000000004, 50.400000000000006, 54.0, 57.6, 61.2, 64.8, 68.4, 72.0, 75.6, 79.2, 82.8, 86.39999999999999, 90.0, 93.60000000000001, 97.2, 100.80000000000001, 104.39999999999999, 108.0, 111.6, 115.2, 118.80000000000001, 122.4, 126.00000000000001, 129.6, 133.2, 136.8, 140.4, 144.0, 147.60000000000002, 151.2, 154.8, 158.4, 162.0, 165.6, 169.20000000000002, 172.79999999999998, 176.4, 180.0, 183.6, 187.20000000000002, 190.8, 194.4, 198.00000000000003, 201.60000000000002, 205.20000000000002, 208.79999999999998, 212.39999999999998, 216.0, 219.6, 223.2, 226.8, 230.4, 234.0, 237.60000000000002, 241.20000000000002, 244.8, 248.40000000000003, 252.00000000000003, 255.6, 259.2, 262.8, 266.4, 270.0, 273.6, 277.2, 280.8, 284.40000000000003, 288.0, 291.6, 295.20000000000005, 298.8, 302.4, 306.0, 309.6, 313.2, 316.8, 320.4, 324.0, 327.6, 331.2, 334.8, 338.40000000000003, 342.0, 345.59999999999997, 349.2, 352.8, 356.4], [-3.4129345079198394, -3.3412517080838695, -3.237842880709583, -3.0973083360014426, -2.9859166836535187, -2.829320175768431, -2.669236171546384, -2.5129432316989937, -2.3121533464653394, -2.0759841318383003, -1.8739589188667278, -1.6777946807306292, -1.35908707268056, -1.0636388397283245, -0.8181649477408169, -0.5448424619494378, -0.268810938572507, -0.06817221457678806, 0.12280208595714834, 0.3068990118243837, 0.5176728122974912, 0.7640484214654104, 1.1419892242071963, 1.4764874111731627, 1.7687536655537712, 1.9923856370582802, 2.230489518034254, 2.392582015741923, 2.628310624570555, 2.8839921952249865, 3.0646199857375125, 3.228820917575184, 3.418900186101924, 3.605506247289413, 3.761202245800331, 3.934731454769414, 4.138446710306242, 4.203446627255555, 4.393742716985177, 4.554280105705182, 4.661203118863906, 4.722655432566134, 4.842692788862879, 4.975328375827054, 5.0250816357838035, 5.0235879877456755, 5.03199804874651, 5.10955641407199, 5.076422708891909, 5.081165639043932, 5.073294825930726, 4.978420708450514, 4.876680272642288, 4.831422684466524, 4.50576833302911, 4.417212643554925, 4.293981334569766, 4.0573348255811705, 3.8308223055333523, 3.6781826302092555, 3.3992040662907965, 3.098348171446738, 2.7759677647358965, 2.6532288821968333, 2.2087811245385116, 2.0747641403735777, 1.7028752593793877, 1.3397681295677217, 1.1989068166427646, 0.9056608299305918, 0.566414893717426, 0.23825842112842593, 0.03867685700082338, -0.2935295463634631, -0.4957018494305457, -0.8266893065380204, -0.9346983965154295, -1.0814553938424425, -1.415773800524059, -1.6424938385879915, -1.8645526799124745, -2.1283812147708008, -2.3065186480997393, -2.534482586698385, -2.7137871545514494, -2.749111980203364, -2.963901950097321, -3.0404420713212703, -3.171244457114342, -3.32857397172566, -3.389054534142446, -3.3978108505400577, -3.505619263216504, -3.518149043494506, -3.594853887191462, -3.6085898408852084, -3.531220620320301, -3.573905680624593, -3.5261637842807394, -3.513813985160611]}
  in  "Plot Channel":u16(ring) items=["LDA (U)", "Gen (Vin)"]
  in  "Plot Data":T3
  out "Phase":T4(graph)
  out "fk":dbl[](array[numeric])
  out "phiK":dbl[](array[numeric])
  out "Ak":dbl[](array[numeric])
  out "Amp":T4(graph)
  in  "index":i32
  out "XY Graph":cluster{"Ramp Pattern":dbl[], "X":dbl[]}(graph)
  out "Data Points":i32[][](array[numeric])=[[1358, 1345, 1296, 1279, 1181, 1241, 1218, 1082, 1071, 960, 945, 848, 827, 742, 747, 751, 677, 739, 745, 766, 766, 737, 764, 790, 872, 945, 1003, 1066, 1169, 1174, 1250, 1309, 1280, 1388, 1423, 1525, 1537, 1567, 1651, 1571, 1663, 1750, 1677, 1743, 1772, 1705, 1797, 1760, 1746, 1725, 1725, 1747, 1685, 1690, 1563, 1571, 1574, 1487, 1458, 1301, 1305, 1275, 1247, 1196, 1110, 1139, 1029, 969, 995, 960, 948, 839, 925, 938, 862, 860, 943, 895, 990, 971, 984, 1037, 1058, 1109, 1122, 1164, 1278, 1226, 1300, 1339, 1395, 1341, 1435, 1376, 1395, 1372, 1444, 1337, 1357, 1373], [1147, 1108, 1116, 1075, 1046, 958, 984, 885, 882, 753, 768, 693, 636, 559, 548, 565, 563, 574, 560, 596, 594, 638, 613, 636, 694, 743, 822, 895, 958, 1079, 1079, 1156, 1163, 1207, 1247, 1248, 1289, 1304, 1365, 1443, 1428, 1457, 1436, 1501, 1564, 1476, 1494, 1421, 1495, 1460, 1460, 1447, 1439, 1424, 1392, 1304, 1278, 1228, 1237, 1132, 1047, 985, 968, 932, 908, 819, 819, 753, 702, 627, 641, 648, 609, 630, 643, 665, 682, 724, 722, 764, 788, 784, 821, 842, 888, 918, 937, 1005, 1043, 1079, 1132, 1099, 1179, 1079, 1153, 1158, 1160, 1177, 1142, 1156], [1604, 1604, 1600, 1600, 1600, 1608, 1600, 1600, 1600, 1604, 1604, 1604, 1596, 1604, 1600, 1600, 1604, 1600, 1600, 1600, 1604, 1600, 1600, 1604, 1596, 1604, 1604, 1600, 1600, 1600, 1596, 1604, 1592, 1596, 1608, 1600, 1600, 1604, 1596, 1604, 1604, 1600, 1596, 1604, 1604, 1600, 1600, 1600, 1600, 1608, 1596, 1600, 1604, 1600, 1604, 1600, 1596, 1604, 1604, 1600, 1596, 1604, 1600, 1600, 1600, 1596, 1596, 1604, 1600, 1604, 1600, 1596, 1604, 1604, 1600, 1604, 1596, 1600, 1608, 1600, 1596, 1600, 1604, 1604, 1600, 1600, 1596, 1608, 1604, 1596, 1600, 1600, 1604, 1608, 1592, 1600, 1604, 1596, 1596, 1600], [1604, 1604, 1600, 1600, 1600, 1608, 1600, 1600, 1600, 1604, 1604, 1604, 1596, 1604, 1600, 1600, 1604, 1600, 1600, 1600, 1604, 1600, 1600, 1604, 1596, 1604, 1604, 1600, 1600, 1600, 1596, 1604, 1592, 1596, 1608, 1600, 1600, 1604, 1596, 1604, 1604, 1600, 1596, 1604, 1604, 1600, 1600, 1600, 1600, 1608, 1596, 1600, 1604, 1600, 1604, 1600, 1596, 1604, 1604, 1600, 1596, 1604, 1600, 1600, 1600, 1596, 1596, 1604, 1600, 1604, 1600, 1596, 1604, 1604, 1600, 1604, 1596, 1600, 1608, 1600, 1596, 1600, 1604, 1604, 1600, 1600, 1596, 1608, 1604, 1596, 1600, 1600, 1604, 1608, 1592, 1600, 1604, 1596, 1596, 1600], [1604, 1604, 1600, 1600, 1600, 1608, 1600, 1600, 1600, 1604, 1604, 1604, 1596, 1604, 1600, 1600, 1604, 1600, 1600, 1600, 1604, 1600, 1600, 1604, 1596, 1604, 1604, 1600, 1600, 1600, 1596, 1604, 1592, 1596, 1608, 1600, 1600, 1604, 1596, 1604, 1604, 1600, 1596, 1604, 1604, 1600, 1600, 1600, 1600, 1608, 1596, 1600, 1604, 1600, 1604, 1600, 1596, 1604, 1604, 1600, 1596, 1604, 1600, 1600, 1600, 1596, 1596, 1604, 1600, 1604, 1600, 1596, 1604, 1604, 1600, 1604, 1596, 1600, 1608, 1600, 1596, 1600, 1604, 1604, 1600, 1600, 1596, 1608, 1604, 1596, 1600, 1600, 1604, 1608, 1592, 1600, 1604, 1596, 1596, 1600], [1604, 1604, 1600, 1600, 1600, 1608, 1600, 1600, 1600, 1604, 1604, 1604, 1596, 1604, 1600, 1600, 1604, 1600, 1600, 1600, 1604, 1600, 1600, 1604, 1596, 1604, 1604, 1600, 1600, 1600, 1596, 1604, 1592, 1596, 1608, 1600, 1600, 1604, 1596, 1604, 1604, 1600, 1596, 1604, 1604, 1600, 1600, 1600, 1600, 1608, 1596, 1600, 1604, 1600, 1604, 1600, 1596, 1604, 1604, 1600, 1596, 1604, 1600, 1600, 1600, 1596, 1596, 1604, 1600, 1604, 1600, 1596, 1604, 1604, 1600, 1604, 1596, 1600, 1608, 1600, 1596, 1600, 1604, 1604, 1600, 1600, 1596, 1608, 1604, 1596, 1600, 1600, 1604, 1608, 1592, 1600, 1604, 1596, 1596, 1600]]
  out "U":dbl[][](array[numeric])=[[-3.4129345079198394, -3.3412517080838695, -3.237842880709583, -3.0973083360014426, -2.9859166836535187, -2.829320175768431, -2.669236171546384, -2.5129432316989937, -2.3121533464653394, -2.0759841318383003, -1.8739589188667278, -1.6777946807306292, -1.35908707268056, -1.0636388397283245, -0.8181649477408169, -0.5448424619494378, -0.268810938572507, -0.06817221457678806, 0.12280208595714834, 0.3068990118243837, 0.5176728122974912, 0.7640484214654104, 1.1419892242071963, 1.4764874111731627, 1.7687536655537712, 1.9923856370582802, 2.230489518034254, 2.392582015741923, 2.628310624570555, 2.8839921952249865, 3.0646199857375125, 3.228820917575184, 3.418900186101924, 3.605506247289413, 3.761202245800331, 3.934731454769414, 4.138446710306242, 4.203446627255555, 4.393742716985177, 4.554280105705182, 4.661203118863906, 4.722655432566134, 4.842692788862879, 4.975328375827054, 5.0250816357838035, 5.0235879877456755, 5.03199804874651, 5.10955641407199, 5.076422708891909, 5.081165639043932, 5.073294825930726, 4.978420708450514, 4.876680272642288, 4.831422684466524, 4.50576833302911, 4.417212643554925, 4.293981334569766, 4.0573348255811705, 3.8308223055333523, 3.6781826302092555, 3.3992040662907965, 3.098348171446738, 2.7759677647358965, 2.6532288821968333, 2.2087811245385116, 2.0747641403735777, 1.7028752593793877, 1.3397681295677217, 1.1989068166427646, 0.9056608299305918, 0.566414893717426, 0.23825842112842593, 0.03867685700082338, -0.2935295463634631, -0.4957018494305457, -0.8266893065380204, -0.9346983965154295, -1.0814553938424425, -1.415773800524059, -1.6424938385879915, -1.8645526799124745, -2.1283812147708008, -2.3065186480997393, -2.534482586698385, -2.7137871545514494, -2.749111980203364, -2.963901950097321, -3.0404420713212703, -3.171244457114342, -3.32857397172566, -3.389054534142446, -3.3978108505400577, -3.505619263216504, -3.518149043494506, -3.594853887191462, -3.6085898408852084, -3.531220620320301, -3.573905680624593, -3.5261637842807394, -3.513813985160611], [-0.4200077572758023, -0.44122827096431866, -0.3944658943656522, -0.3820905317351646, -0.3698483905061325, -0.3638499115795391, -0.32118280802234306, -0.26788959486721575, -0.2847754693783302, -0.27076915178956684, -0.23596601346602158, -0.1719737076329121, -0.11105845083008924, -0.10693828209479256, -0.1314447121913005, -0.06972850200284014, -0.046887857505642776, 0.007659514184652489, -0.021349734118240895, 0.04144638883914862, 0.05606558235447396, 0.04225561481117978, 0.10821331077099833, 0.15516669394235932, 0.2155867569402253, 0.19231561270907652, 0.2274845581183134, 0.2773367551175649, 0.28881659329074266, 0.35053904097800165, 0.36086570353378916, 0.37601689142292555, 0.4041702508222837, 0.4237384007649119, 0.45733906624148596, 0.4835740044215842, 0.5481346016230898, 0.5007426915621356, 0.575116281989454, 0.6382748411454698, 0.6601989577764749, 0.6577630455843821, 0.7244856394337288, 0.6532193010850835, 0.727736737694325, 0.6650632723502117, 0.692857274655635, 0.6619417747174531, 0.6487970023530039, 0.6231932686547025, 0.6466189985093068, 0.575112204900599, 0.556917730491972, 0.49598747446508035, 0.41087006821181205, 0.3918854163951234, 0.2807392097637791, 0.2905321980236355, 0.18724463465214355, 0.17981855183513235, 0.08755003783346924, 0.06519640409075843, 0.003541818855763959, -0.11109594662500463, -0.0483164279544499, -0.18565708979530926, -0.2500913845936301, -0.22861507939314826, -0.31697840270432426, -0.3915062888113033, -0.3000021311744795, -0.4109490116601009, -0.4756574473200575, -0.48044372217559744, -0.43227319853806345, -0.5283948081043567, -0.4756382149226868, -0.44947778392975535, -0.5767359467907794, -0.5693798580688151, -0.6066279533891391, -0.6553942991791939, -0.6638443233951395, -0.675220763542928, -0.6611183444056463, -0.6642068588104594, -0.7069207780145301, -0.653478158968213, -0.635750770690451, -0.6581257987398099, -0.6234387598807544, -0.5640364112119536, -0.6368127164654787, -0.5557784184821881, -0.5650258884387831, -0.5186154761289171, -0.5036148310160348, -0.4676922863719135, -0.4789670190451544, -0.5182694199025035], [-0.005962902694880684, -0.006994368922434381, -0.007982647326339253, -0.008952951067038467, -0.009886522844645007, -0.0107712369481883, -0.011628812570022651, -0.012440617315110522, -0.013185022425456439, -0.013904903014172984, -0.014547519214842338, -0.01514436551381067, -0.015687943562685033, -0.016154989146964296, -0.016578223379467974, -0.01692247367002136, -0.017211318920218363, -0.017428806256617017, -0.017576140516193446, -0.017662159852169724, -0.017678492661363964, -0.01762538759811633, -0.017506366164460885, -0.017314843754799858, -0.017067013708882448, -0.016743423820744712, -0.016357842579071597, -0.015912128036733923, -0.015398712599936037, -0.014839895754282932, -0.01421793817979229, -0.013535418536864737, -0.012803137447939308, -0.012029993107670407, -0.011202587538294147, -0.010327029582384444, -0.0094311005277015, -0.008463823396508606, -0.007476842346596942, -0.006482463020748315, -0.005443711142384791, -0.004397392716641737, -0.0033139656957754436, -0.0022405405874115453, -0.0011458434682604316, -5.676101495210684e-05, 0.0010169217502451978, 0.0021342937040094083, 0.0031935061916661396, 0.00425924750324462, 0.005295387100905992, 0.006311408026740565, 0.007318864265531032, 0.008279819948471545, 0.009201748252679946, 0.01008358718446156, 0.010938221993257441, 0.011739374167533326, 0.012499381748239896, 0.0132018237437582, 0.013851931801580524, 0.014449155964147583, 0.014985930905004637, 0.01546775714331108, 0.015874947541419205, 0.016236099598561506, 0.01651542785385255, 0.01673447682048175, 0.016894511352264507, 0.016982252890078032, 0.01700008018642851, 0.016955944379090218, 0.016835787302930668, 0.016649085377386554, 0.016398964031171966, 0.016079980302611447, 0.015695729483424833, 0.015250210423183507, 0.014735695019741306, 0.014164977612851104, 0.013545598266756935, 0.012859825569554301, 0.012129991637925212, 0.011338767422211345, 0.010509699047922347, 0.009632927593870029, 0.008722522868845374, 0.0077786491575999265, 0.006780400200590205, 0.005787595402689878, 0.004734620221388978, 0.0036982570728058563, 0.0026305167211487343, 0.001531302004332368, 0.0004500415508618359, -0.0006447174255391533, -0.001725522709132289, -0.0027892743560575537, -0.003871284031843999, -0.004949987820056926], [-0.0509787667975431, -0.05100587356289877, -0.05078987625575489, -0.050378476591344805, -0.04972909618612768, -0.04888595361760317, -0.04779927959174752, -0.04647419889381447, -0.04496357817406373, -0.043174801224050874, -0.041227358622000464, -0.039057214617736986, -0.03669758402263296, -0.034163181400718404, -0.03142702727876219, -0.028611551433385986, -0.025565720213430797, -0.022520728253937444, -0.019312899372669813, -0.01603929035800743, -0.012741083723239484, -0.009317823799948301, -0.005979229220472847, -0.0025563897705476665, 0.0007282828070610503, 0.004080533977376609, 0.007298593012349358, 0.010479664816927782, 0.013636045089129982, 0.016631276696136364, 0.01958213587008714, 0.02249906973549201, 0.02530668251974238, 0.02805931480746552, 0.030680962107608185, 0.03326810578784354, 0.03571607650248342, 0.038126771247251175, 0.04037003003979453, 0.04244089442292334, 0.044391369801227445, 0.046152783070721855, 0.0477569753332945, 0.049126647712245744, 0.05028287402626065, 0.051248118429350314, 0.05196435495698812, 0.0524523000245258, 0.052685373690786276, 0.05265271166100886, 0.0524148481280048, 0.051885965917114564, 0.05111565494367806, 0.050118126039086455, 0.048886685427354026, 0.047467272371439356, 0.04578510886389001, 0.04392787662471011, 0.04189168255150877, 0.03966177921021683, 0.0372934509550833, 0.03473683479289667, 0.032077405047019635, 0.02927467035433434, 0.026429149300066727, 0.02335727642764006, 0.020387172606101293, 0.01729771668233603, 0.014132807152022663, 0.011020275309636588, 0.007872891991389989, 0.004808456722277857, 0.001718300789951292, -0.0012865749470842645, -0.004200416734951781, -0.007036359830749954, -0.009852108158482828, -0.012506436265210464, -0.015126438539220508, -0.01767188297654468, -0.020093917909107865, -0.0224826227042666, -0.02479101591382858, -0.027081673389240356, -0.029266432605136554, -0.031441965090207614, -0.03350934411728545, -0.03551387252779318, -0.03747079563052326, -0.039301200229136295, -0.04110990184352959, -0.04270906713842654, -0.04421941076883518, -0.04565115508659845, -0.04693158758609212, -0.048052206985991816, -0.048973410340435064, -0.04975626521917376, -0.050345942966665995, -0.05079320284100726], [233.31913863944476, 295.7666196138201, 356.43097632400065, 416.841725183357, 476.1693241511608, 533.2263534968985, 589.6425307198978, 644.1571289513087, 694.9690534030133, 745.015622847154, 790.2346676148278, 832.9926324877648, 872.1531952720655, 905.9316635827481, 936.883878648928, 962.4174594438359, 983.9907936122244, 1001.1142005214825, 1013.7440961634751, 1022.7228952372775, 1028.068263430813, 1029.9197800082902, 1028.4324033316122, 1023.7579742661732, 1016.2765441054033, 1005.4937053022918, 991.5660739591812, 974.7523525436112, 954.2995022088226, 930.9915465521827, 903.9745689948525, 872.6980814955399, 837.718719522524, 799.2198484596139, 756.2808767693805, 709.3526277177523, 659.7972998419957, 604.6709178362653, 547.3918474363768, 488.4306713761988, 425.9622598878816, 362.6083809981693, 296.3825161891939, 230.57140307379154, 163.48557700126563, 96.72130267039263, 31.15355533703645, -37.022099169672785, -101.54428814244818, -166.6121406413338, -230.55212712698537, -293.58612285590465, -357.281706482234, -419.1712328944718, -480.08265982244353, -540.0106335248538, -599.6724113984762, -657.2904359684147, -713.2837237749551, -766.300971105097, -816.4400960107125, -863.6212742710151, -906.5507960155502, -945.7429744025004, -979.3390324414705, -1009.6652298157944, -1033.8093274747184, -1053.6607775929501, -1069.4377972988673, -1080.2144122849063, -1086.289677286184, -1088.667563683974, -1086.6703512114022, -1080.9290414163988, -1071.7879896299971, -1058.7095356044442, -1042.4228198010408, -1022.3562538504158, -998.1887582860686, -970.8407229292478, -939.6361379258018, -904.0548717996577, -864.8512440343724, -820.6345123834446, -773.0939023370306, -720.9904194729793, -665.7045660425551, -607.1388836503871, -544.375281125654, -481.7204766441207, -415.20675764118937, -349.77883658511564, -283.32154879573585, -215.46730217935706, -149.51305461670353, -83.71804778293743, -19.12866726373699, 44.07338562441554, 108.2869140546797, 172.45936087272344], [-0.04834149322919361, -0.048826267502530954, -0.04922303924523851, -0.04944544382352849, -0.04952823310572497, -0.04945985084440588, -0.04937487163219172, -0.04929281633854434, -0.04902045404829708, -0.04862385268338215, -0.0481950018816458, -0.04769458473609845, -0.047117911047507385, -0.04641223841658145, -0.04571380430012148, -0.04491232192683493, -0.04398942157320853, -0.042938966583009865, -0.04186015874276201, -0.040718009559863315, -0.03938818242017179, -0.03788600472877459, -0.03634447882601438, -0.03457730500416773, -0.032887081424998486, -0.030898441001134976, -0.028842539653276277, -0.026611322319007175, -0.024284750569074993, -0.022043921893517546, -0.019403489431814813, -0.016788061877512042, -0.014002426490840046, -0.011157595940547839, -0.008314114358740878, -0.005276847006417193, -0.0023303521787374844, 0.000715421795541856, 0.003785663593693458, 0.006751945301473301, 0.009645780692552492, 0.012543497930926168, 0.015453066757985566, 0.01818879716591558, 0.020753468758379526, 0.023294426600339837, 0.0256729125505174, 0.028031917125095663, 0.030117811252542367, 0.03224535092501938, 0.03409443945239982, 0.03572697201080891, 0.03720942407118591, 0.03856741852772935, 0.03965425416698299, 0.040567069488709084, 0.041181930971348646, 0.041563713380444296, 0.04185783741756318, 0.04179008218633424, 0.04150205235999115, 0.04110479353267937, 0.04030154729946087, 0.039396318299764185, 0.03820576751273708, 0.036779852868817624, 0.03499505098055045, 0.03325391503634546, 0.031242751485187226, 0.02879761750227364, 0.02634239945968345, 0.023723802454039895, 0.02096775038311346, 0.017965046912596094, 0.014908221358500841, 0.0116473262582104, 0.008402284288829142, 0.005035807889193075, 0.0016500399189746974, -0.0018478181989211126, -0.005167677785313819, -0.008593345526108609, -0.011830662858787037, -0.015087925467352601, -0.018206384056245643, -0.02131115454246944, -0.02419564958171643, -0.026852761203173564, -0.029552918716782405, -0.031999815442541116, -0.03436695449466149, -0.036508539302147314, -0.03853847492725914, -0.04043348452509024, -0.04206323081330674, -0.04356116613080804, -0.04481974003229292, -0.04598211956784874, -0.04680931918833959, -0.04774898307364484]]
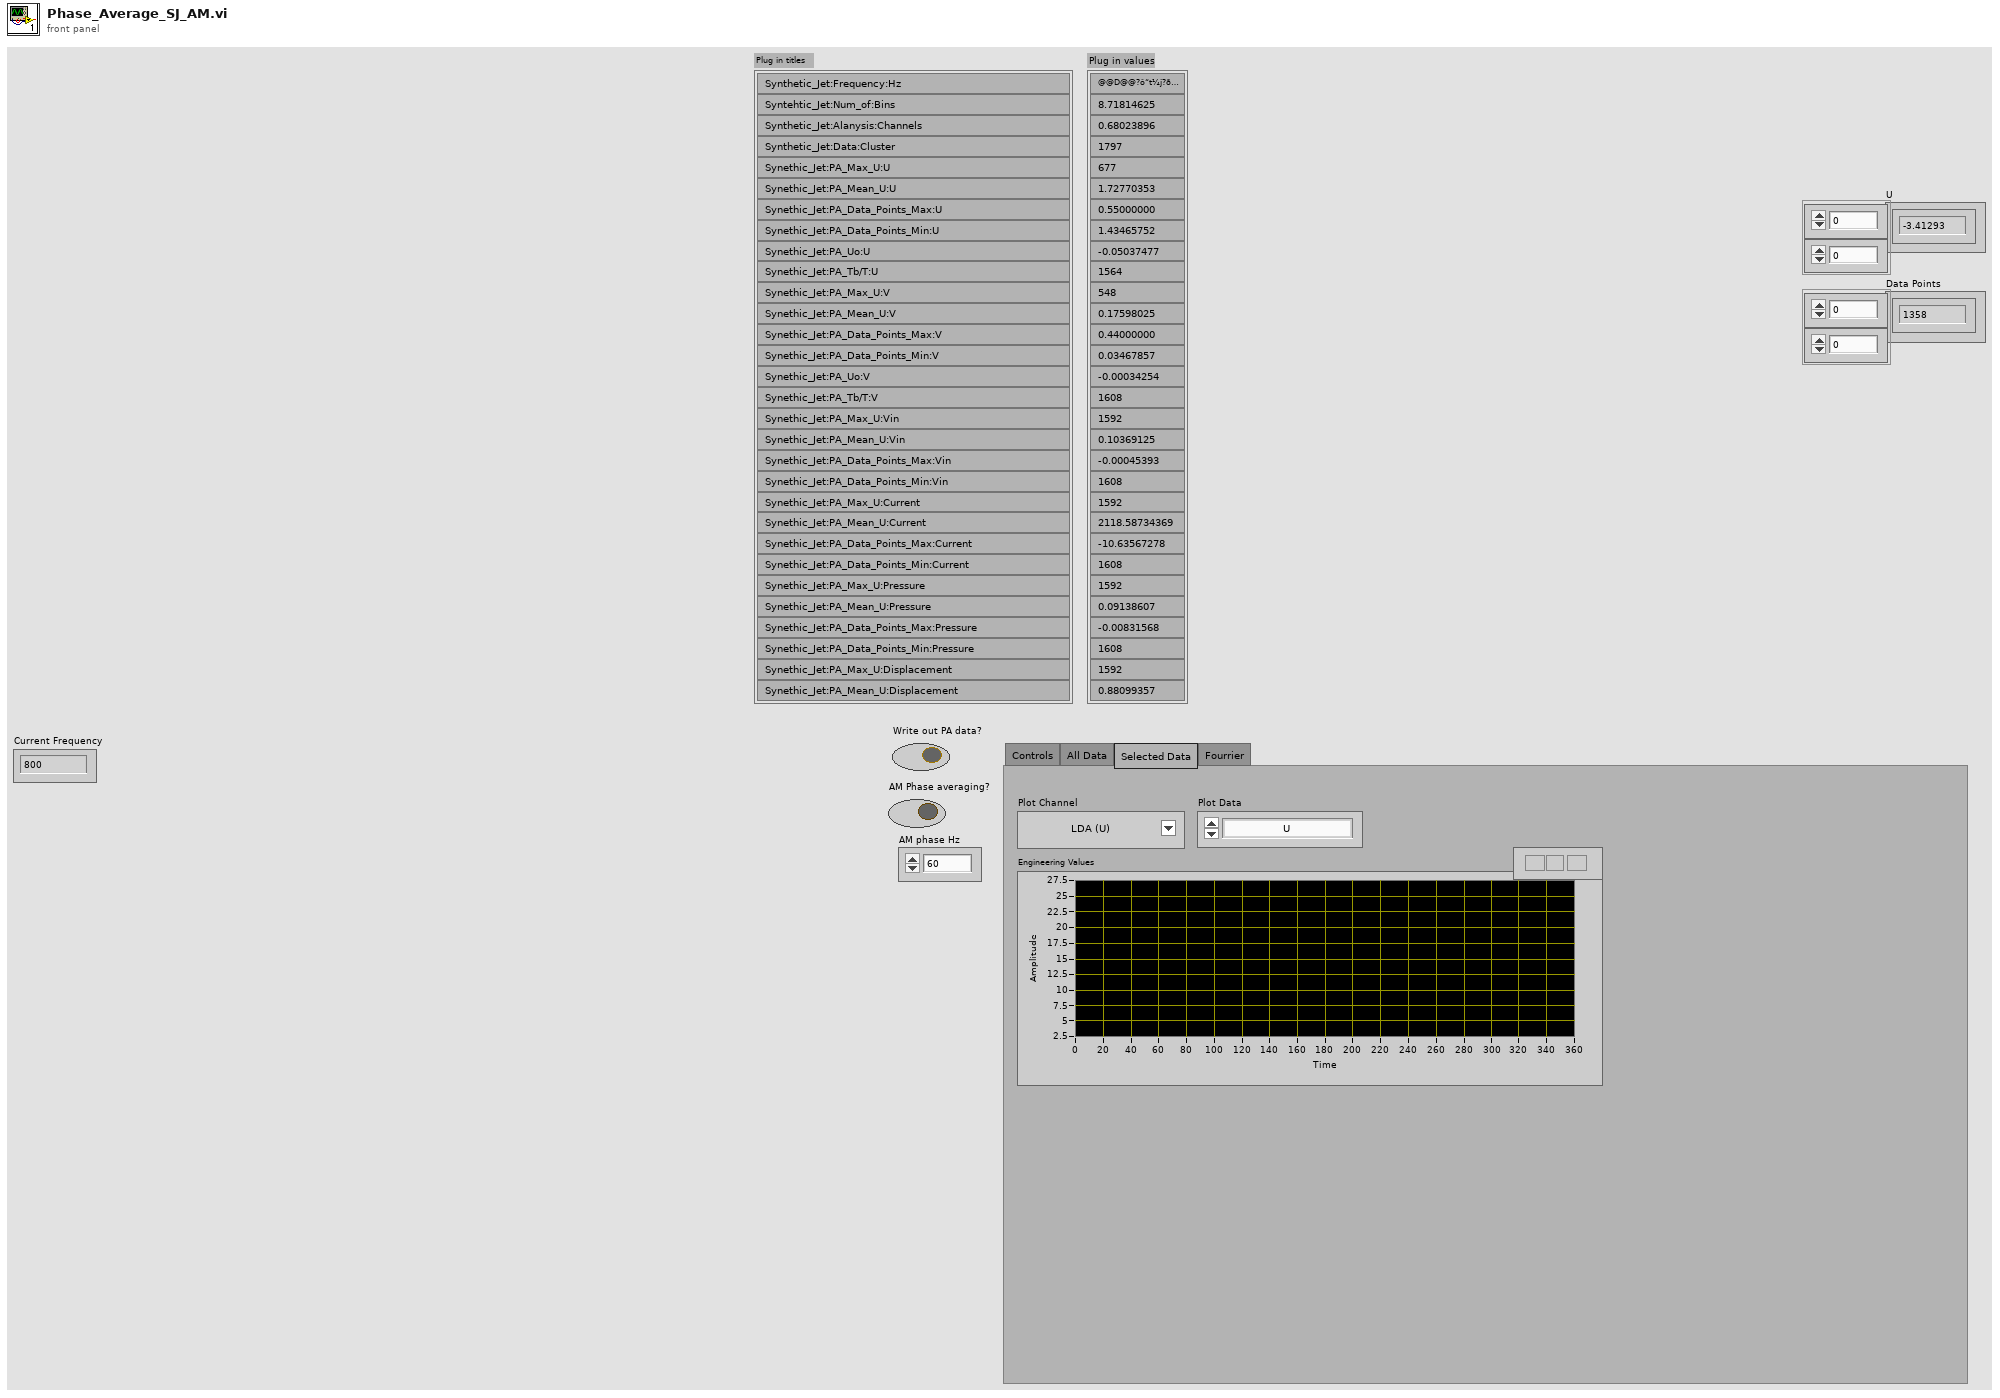
[diagram p1: front panel]
types:
  T1 = enum32{"Controls", "All Data", "Selected Data", "Fourrier"}
  T2 = typedef "SJ_Data_Cluster.ctl" = cluster{"Do (mm)":dbl, "Dc (mm)":dbl, "Ho (mm)":dbl, "Hc (mm)":dbl, "K":dbl, "beta":dbl, "Vc (m^3)":dbl, "Vo (m^3)":dbl}
  T3 = typedef "Stats_Menu.ctl" = enum16{"U", "u^2", "u^3", "u^4", "Skew_u", "Kurt_u", "% u'/U"}
  T4 = cluster{"Ramp Pattern":dbl[], "Amp Spectrum Mag (Vrms)":dbl[]}
  T5 = typedef "Analysis_info_cluster.ctl" = cluster{"Colour":u32, "Inst type":T6, "Inst name":string, "Symbol":string, "Code name":string, "Extra Info":string, "Inst Array":T7, "Extra Titles":string[], "Extra Values":string[], "U":dbl, "u^2":dbl, "u^3":dbl, "u^4":dbl, "Skew_u":dbl, "Kurt_u":dbl, "Sd Error in Mean":dbl, "% u'/U":dbl, "X":dbl, "Y":dbl, "Z":dbl, "Timescale integral to 25%":dbl, "Sd Error in Variance":dbl, "Calib File":path, "Calib Constants":dbl[], "Output Position":bool, "Full Stats":bool, "Av Sampling Rate":dbl, "Av No of Samples":dbl, "Total Meas Time (s)":dbl, "ADAM Ch Name":string}
  T6 = typedef "Inst_type.ctl" = enum16{"Propeller anemometer", "Raw voltage", "Pressure Transducer", "Pitot-static tube", "Preston tube", "Hot wire", "Cross wire 1", "Cross wire 2", "Generic Linear", "Generic Polynomial", "Generic BackPoly", "Fast FID", "Thermocouple", "Cold wire", "Pulsed Wire", "LDA Vel", "LDA Tran time", "LDA Arr time"}
  T7 = typedef "Instrument_Array.ctl" = enum16{"PWA", "LDA", "Analogue"}
  T8 = typedef "Time_Trace_Cluster.ctl" = cluster{"Weighting":dbl[], "Time (s)":dbl[], "Voltage":dbl[], "Eng Values":dbl[]}
  T9 = typedef "Post_Process.ctl" = enum16{"Take New Data", "Post Process Raw Data File"}
  T10 = enum16{"SJ Data Cluster to String", "String to SJ Data Cluster"}
  T11 = typedef "Bin_Cluster.ctl" = cluster{"Start Time":dbl, "End Time":dbl, "Bin Number":i32, "Data Points":i32, "Shift":dbl[], "Stats":cluster{"U":dbl, "u^2":dbl, "u^3":dbl, "u^4":dbl, "Skew_u":dbl, "Kurt_u":dbl, "% u'/U":dbl}, "Channel Name":string, "Bin Centre":dbl, "Symbol":string}
  T12 = cluster{"Ramp Pattern":dbl[], "Amp Spectrum Phase (radians)":dbl[]}
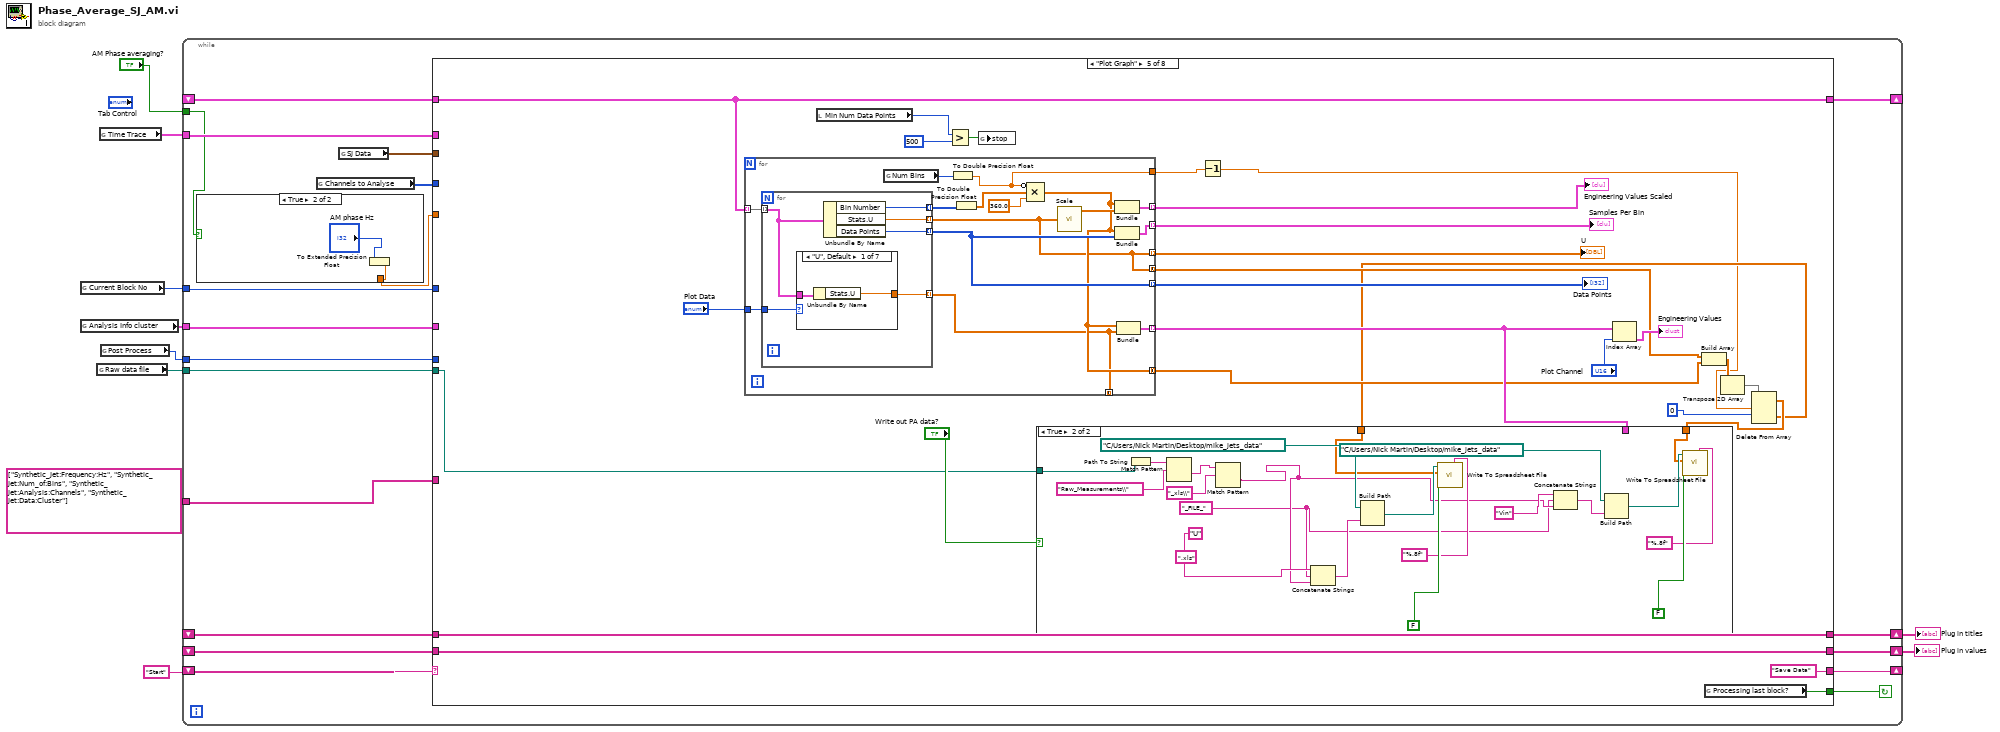
[diagram p0: block diagram]
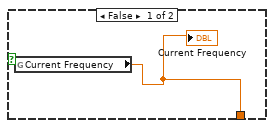
[diagram p2: hidden frame]
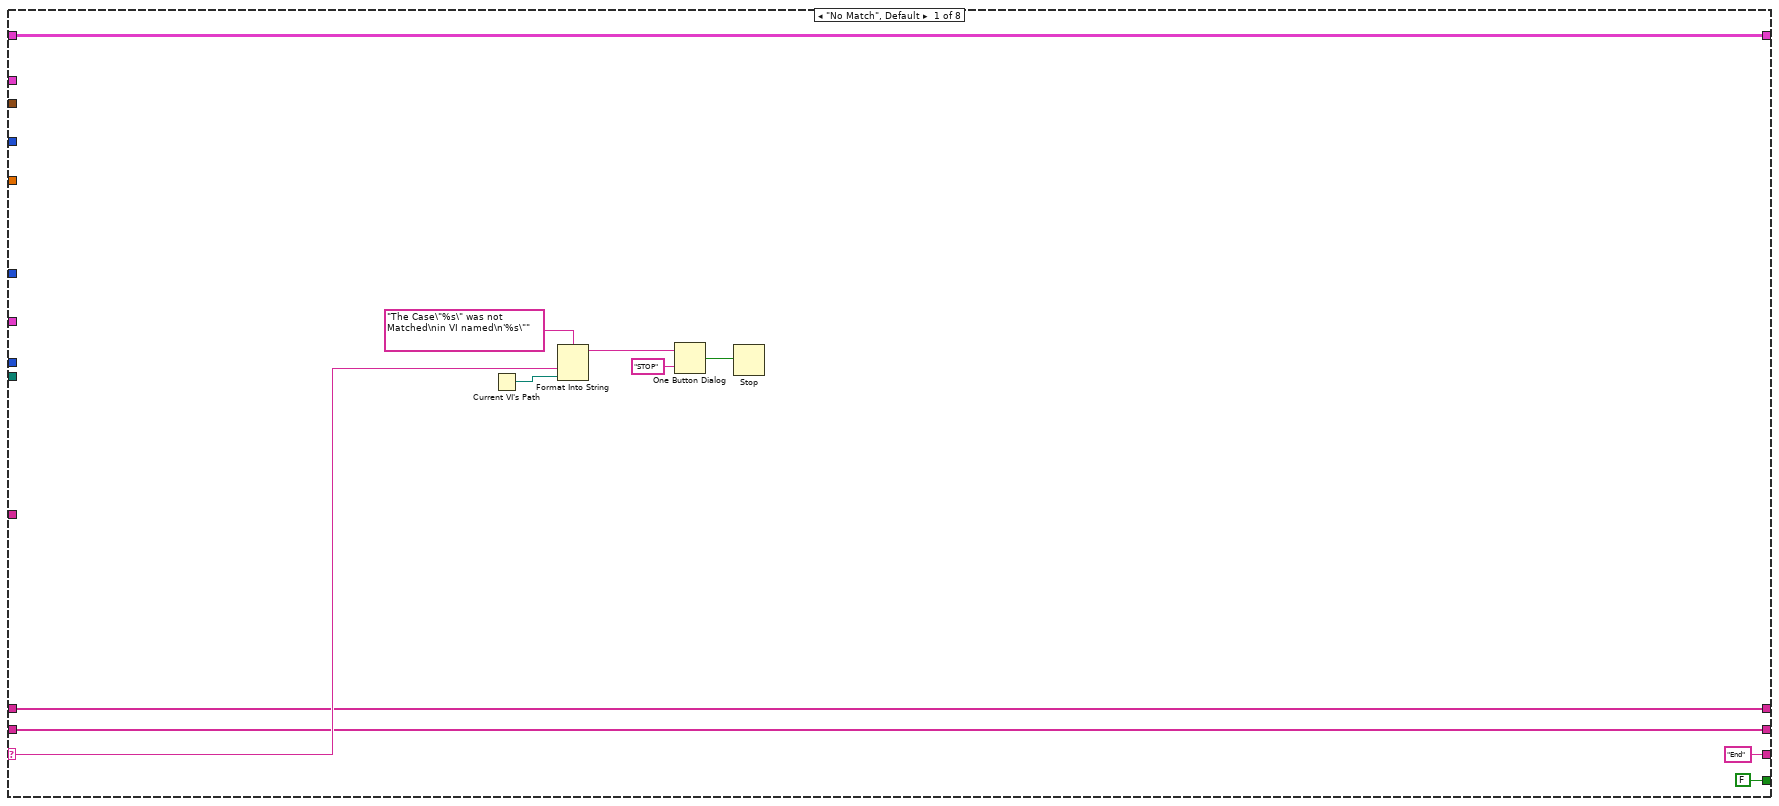
[diagram p3: hidden frame]
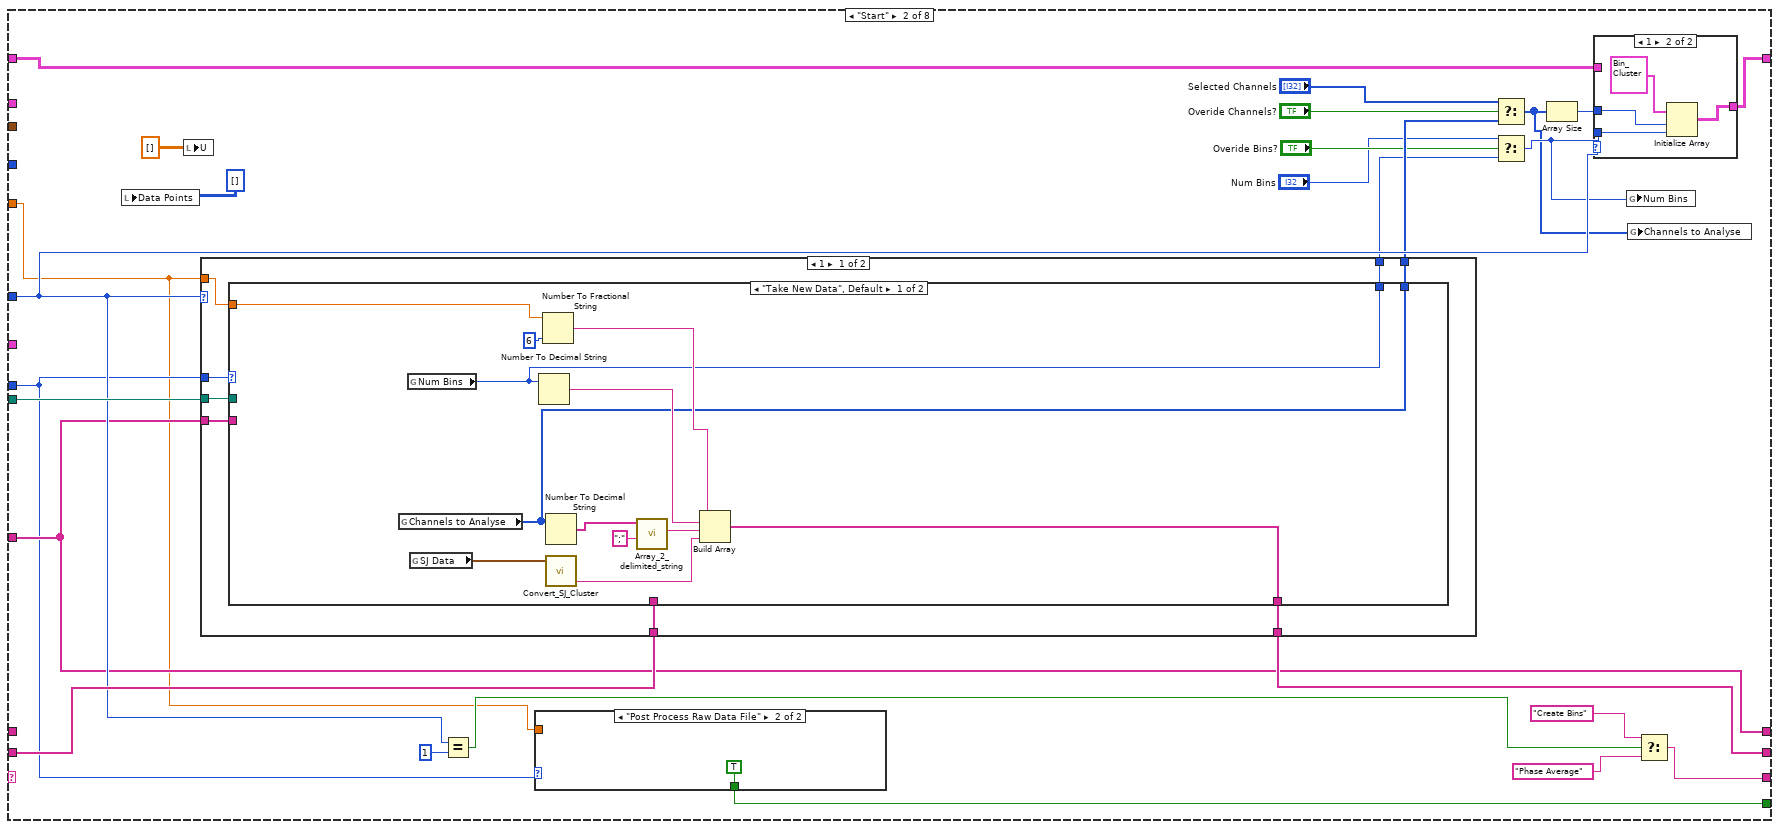
[diagram p4: hidden frame]
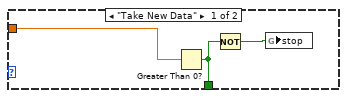
[diagram p5: hidden frame]
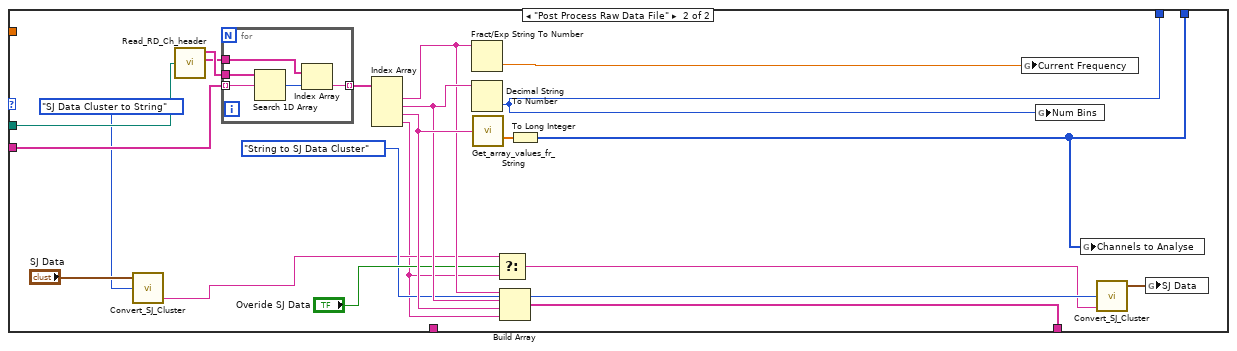
[diagram p6: hidden frame]
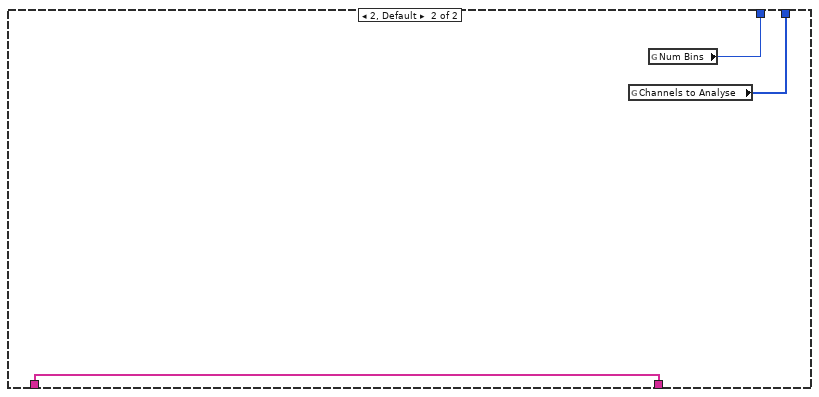
[diagram p7: hidden frame]
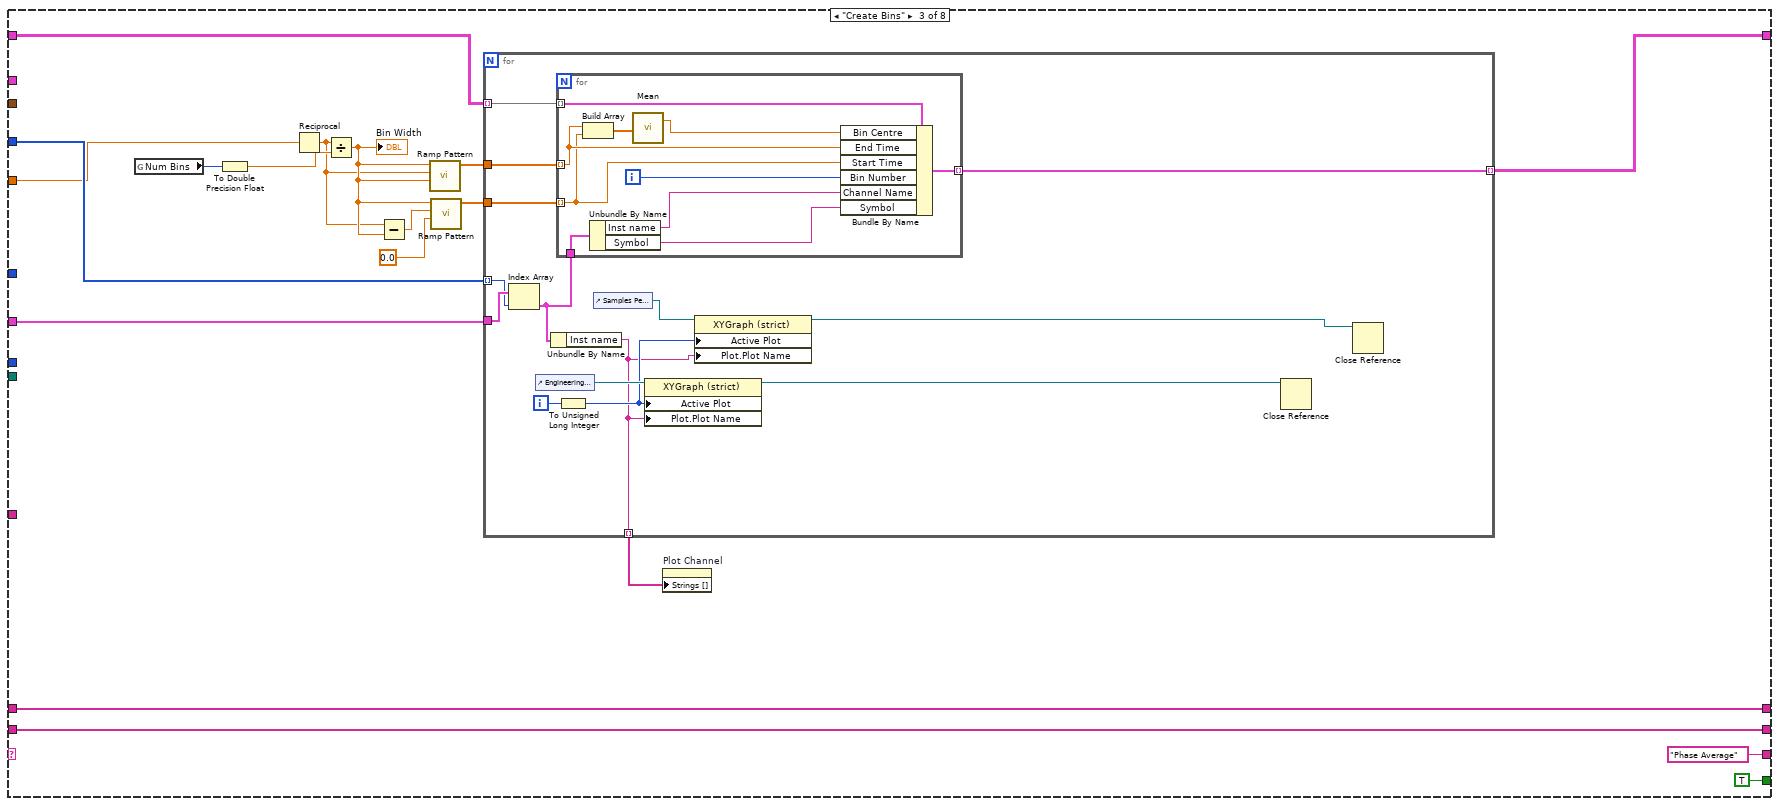
[diagram p9: hidden frame]
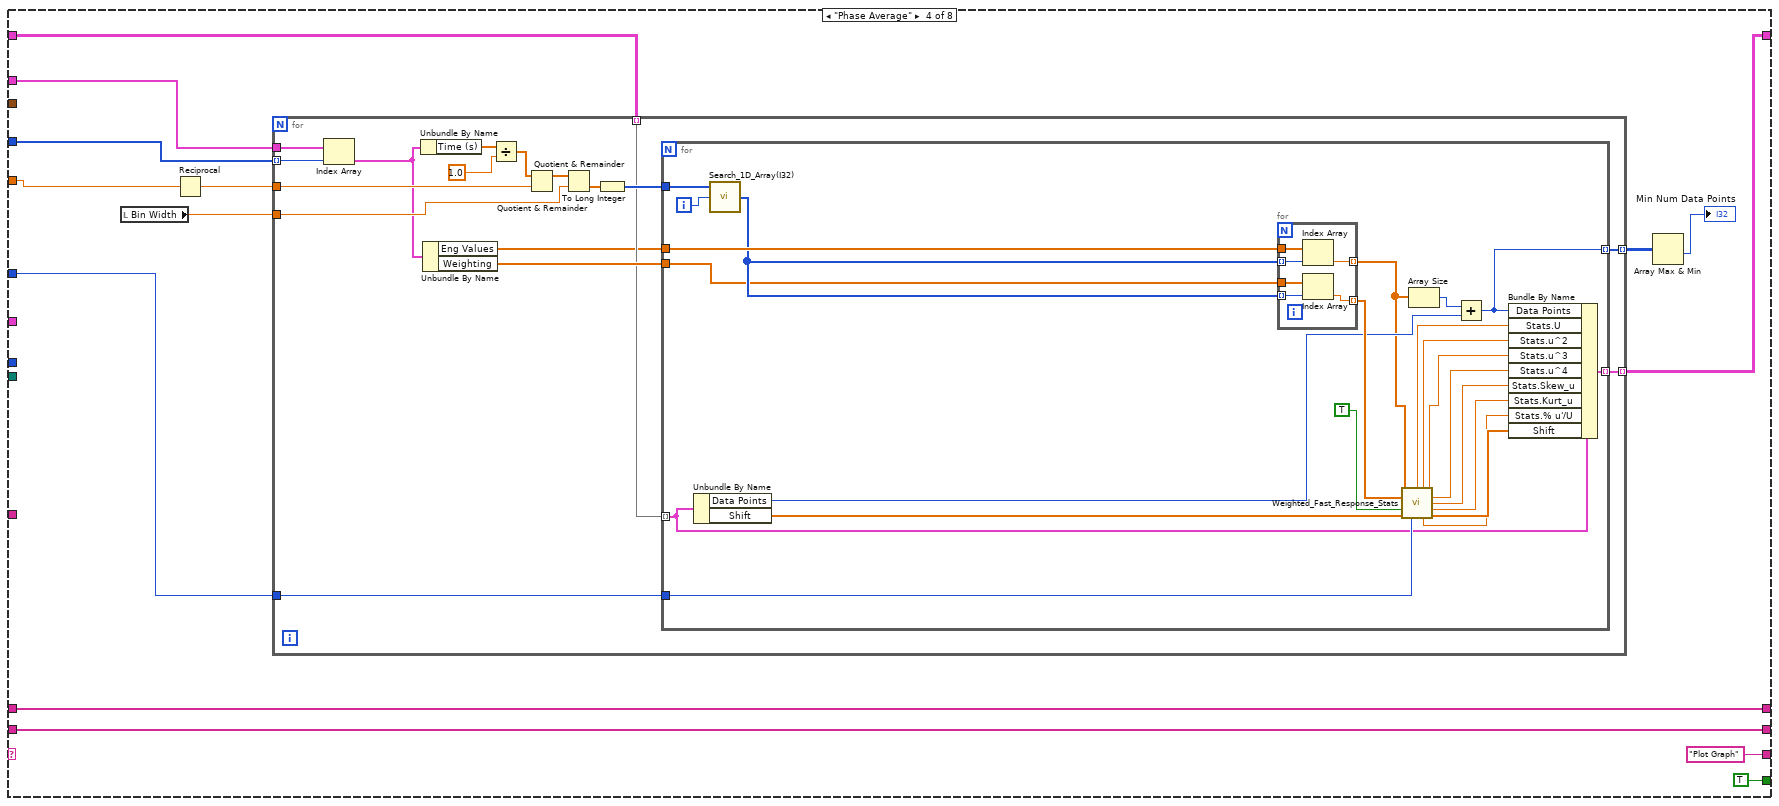
[diagram p10: hidden frame]
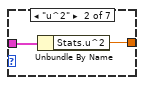
[diagram p12: hidden frame]
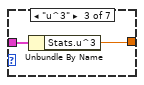
[diagram p13: hidden frame]
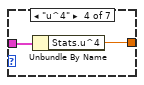
[diagram p14: hidden frame]
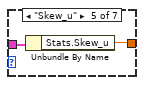
[diagram p15: hidden frame]
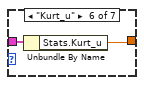
[diagram p16: hidden frame]
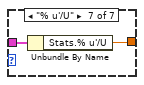
[diagram p17: hidden frame]
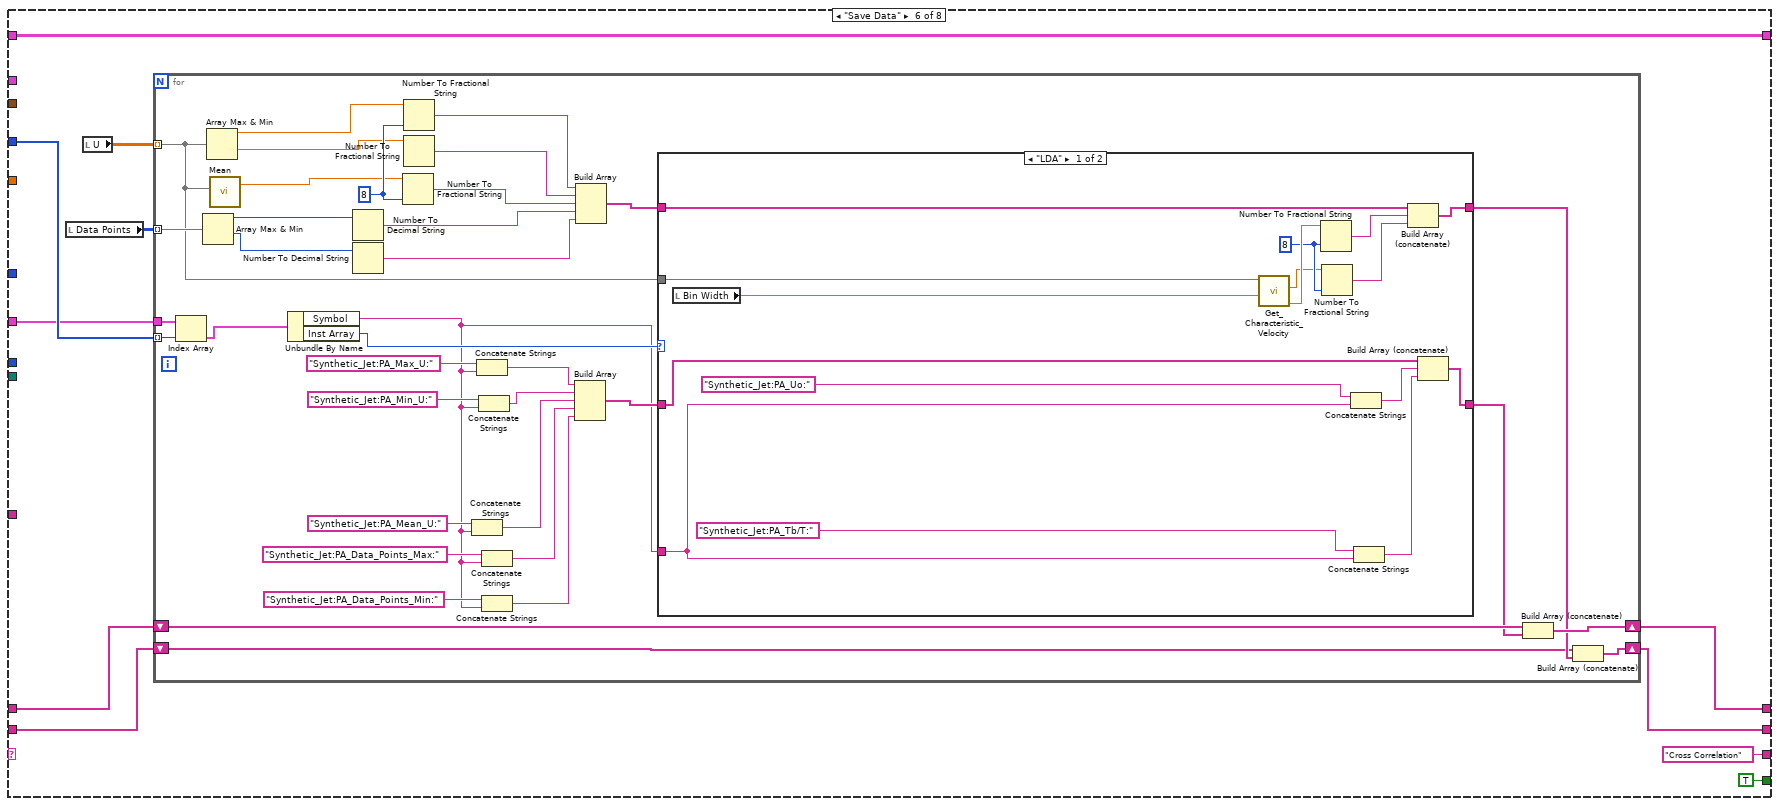
[diagram p18: hidden frame]
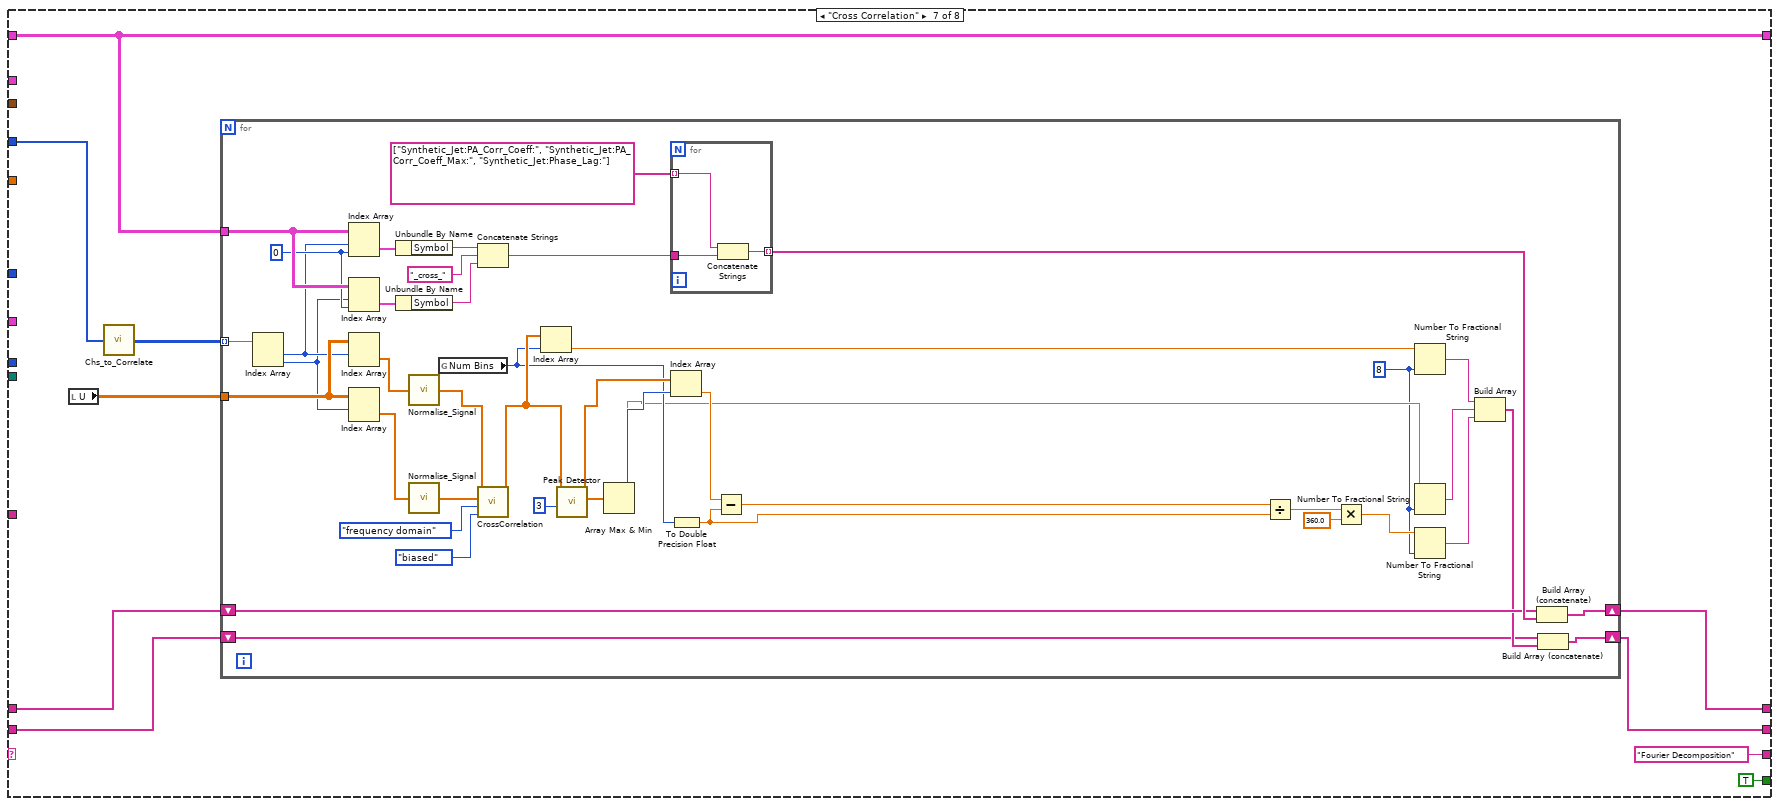
[diagram p20: hidden frame]
diagram:
  n1 = global read "Meas_global.vi" "Current Block No"() -> (w8:i32)
  n2 = global read "Meas_global.vi" "Analysis Info cluster"() -> (w7:T5[])
  n3 = global read "Meas_global.vi" "Raw data file"() -> (w5:path)
  n4 = global read "Meas_global.vi" "Time Trace"() -> (w9:T8[])
  n5 = global read "Meas_global.vi" "Post Process"() -> (w6:T9)
  n6 = while {
    shift-right: [w27] -> _
    shift-left: "Start" -> [w28]
    tunnel: w9 -> [w26]
    shift-right: [w23] -> _
    shift-left: _ -> [w25]
    tunnel: w8 -> [w24]
    tunnel: w7 -> [w22]
    tunnel: w6 -> [w21]
    tunnel: w5 -> [w20]
    shift-right: [w18] -> w4
    shift-left: _ -> [w19]
    shift-right: [w16] -> w3
    shift-left: _ -> [w17]
    tunnel: string[] ["Synthetic_Jet:Frequency:Hz", "Synthetic_Jet:Num_of:Bins", "Synthetic_Jet:Analysis:Channels", "Synthetic_Jet:Data:Cluster"] ("Desired Ch Names") -> [w13]
    tunnel: "AM Phase averaging?" -> [w11]
    stop <- w29 continue-if-true
    n7 = case shown="True" w11 {
      tunnel: [w30 w31] -> w12
      frame False {
        n8 = global read "Synthetic_jet_global.vi" "Current Frequency"() -> (w30:dbl)
        "Current Frequency" <- w30
      }
      frame True {
        n9 = To Extended Precision Float(1:"AM phase Hz") -> (0:w31:ext)
      }
    }
    n10 = global read "Synthetic_jet_global.vi" "Channels to Analyse"() -> (w15:i32[])
    n11 = global read "Synthetic_jet_global.vi" "SJ Data"() -> (w14:T2)
    n12 = case shown="\"Plot Graph\"" w28 {
      selector: w28 -> [w38 _ _ _ _ _ _ _]
      tunnel: [FALSE w46 TRUE TRUE w248 TRUE ("Processing last block?") TRUE ("Processing last block?") FALSE ("Processing last block?")] -> w29
      tunnel: ["End" w62 "Phase Average" "Plot Graph" "Save Data" "Cross Correlation" "Fourier Decomposition" "End"] -> w27
      tunnel: w26 -> [_ _ _ w172 _ _ _ _]
      tunnel: w25 -> [w35 w68 w137 w178 w255 w321 w384 w447]
      tunnel: [w35 w69 w136 w177 w255 w321 w384 w447] -> w23
      tunnel: w24 -> [_ w60 _ w179 _ _ _ _]
      tunnel: w22 -> [_ _ w135 _ _ w313 _ w437]
      tunnel: w21 -> [_ w45 _ _ _ _ _ _]
      tunnel: w20 -> [_ w66 _ _ w230 _ _ _]
      tunnel: [w34 w55 w132 w175 w253 w318 w382 w448] -> w18
      tunnel: w19 -> [w34 _ w132 w175 w253 w319 w383 w449]
      tunnel: [w33 w64 w131 w174 w252 w316 w380 w439] -> w16
      tunnel: w17 -> [w33 w65 w131 w174 w252 w317 w379 w438]
      tunnel: w15 -> [_ _ w130 w171 _ w314 w386 w436]
      tunnel: w14 -> [_ _ _ _ _ _ _ _]
      tunnel: w13 -> [_ w55 _ _ _ _ _ _]
      tunnel: w12 -> [_ w44 w128 w170 _ _ _ w434]
      frame "No Match", Default {
        n13 = Current VI's Path() -> (path=w43:path)
        n14 = Format Into String(format string="The Case\"%s\" was not Matched\nin VI named\n'%s\"" ("Format String"), w38, w43) -> (resulting string=w40:string)  [unwired: 2 in, 1 out]
        n15 = One Button Dialog(message=w40, button name ("OK")="STOP") -> (true=w42:bool)
        n16 = Stop(stop? (T)=w42) -> ()
      }
      frame "Start" {
        n17 = local write "Data Points"(i32[][] [] ("Data Points")) -> ()
        n18 = local write "U"(dbl[][] [] ("U")) -> ()
        n19 = case shown="1" w60 {
          tunnel: w45 -> [w81 _]
          tunnel: [w80 w121] -> w51
          tunnel: [w79 w122] -> w64
          tunnel: w55 -> [w78 _]
          tunnel: w65 -> [w77 w122]
          tunnel: w66 -> [w76 _]
          tunnel: [w75 w120] -> w52
          tunnel: w44 -> [w74 _]
          frame 1 {
            n20 = case shown="\"Take New Data\", Default" w81 {
              tunnel: w78 -> [_ w112]
              tunnel: [w90 w109] -> w80
              tunnel: [w89 w102] -> w79
              tunnel: w77 -> [_ _]
              tunnel: w76 -> [_ w107]
              tunnel: [w83 w101] -> w75
              tunnel: w74 -> [w82 _]
              frame "Take New Data", Default {
                n21 = global read "Synthetic_jet_global.vi" "Channels to Analyse"() -> (w83:i32[])
                n22 = global read "Synthetic_jet_global.vi" "Num Bins"() -> (w90:i32)
                n23 = global read "Synthetic_jet_global.vi" "SJ Data"() -> (w85:T2)
                n24 = Number To Decimal String(number=w90) -> (decimal integer string=w91:string)  [unwired: 1 in]
                n25 = Number To Fractional String(number=w82, precision (6)=i16 6) -> (F-format string=w92:string)  [unwired: 2 in]
                n26 = Number To Decimal String(number=w83) -> (decimal integer string=w88:string[])  [unwired: 1 in]
                n27 = call "Convert_SJ_Cluster.vi"("SJ Data"=w85) -> ("SJ Data String Out"=w84:string)  [unwired: 3 in, 1 out]
                n28 = call "Array_2_delimited_string.vi"("delimiter (Tab)"=";", "Array of Strings"=w88) -> ("delimited string"=w86:string)  [unwired: 9 in]
                n29 = Build Array(w92, w91, w86, w84) -> (w89:string[])
              }
              frame "Post Process Raw Data File" {
                n30 = call "Convert_SJ_Cluster.vi"("Mode"=T10."SJ Data Cluster to String", "SJ Data"="SJ Data") -> ("SJ Data String Out"=w96:string)  [unwired: 2 in, 1 out]
                n31 = call "Read_RD_Ch_header.vi"("Raw data file"=w107) -> ("Ch Name Out"=w114:string[], "Ch Values"=w113:string[])  [unwired: 2 out]
                n32 = for {
                  tunnel: w114 -> [w119]
                  tunnel: w113 -> [w118]
                  tunnel: w112 -> [w116] mode=indexing
                  tunnel: [w115] -> w111 mode=indexing
                  n33 = Search 1D Array(1D array=w119, element=w116) -> (index of element=w117:i32)  [unwired: 1 in]
                  n34 = Index Array(array=w118, index=w117) -> (element=w115:string)
                }
                n35 = Index Array(array=w111) -> (element #1=w103:string, element #2=w104:string, element #3=w105:string, element #4=w94:string)  [unwired: 4 in]
                n36 = Fract/Exp String To Number(string=w103) -> (number=w110:dbl)  [unwired: 3 in, 1 out]
                n37 = Decimal String To Number(string=w104) -> (number=w109:i32)  [unwired: 2 in, 1 out]
                n38 = call "Get_array_values_fr_String.vi"("String Value"=w105) -> ("Numeric Array"=w108:dbl[])  [unwired: 1 out]
                n39 = Select(t=w96, s="Overide SJ Data", f=w94) -> (s? t:f=w95:string)
                n40 = Build Array(w103, w104, w105, w94) -> (w102:string[])
                n41 = To Long Integer(number=w108) -> (32bit integer=w101:i32[])
                n42 = global write "Synthetic_jet_global.vi" "Current Frequency"(w110) -> ()
                n43 = global write "Synthetic_jet_global.vi" "Num Bins"(w109) -> ()
                n44 = global write "Synthetic_jet_global.vi" "Channels to Analyse"(w101) -> ()
                n45 = call "Convert_SJ_Cluster.vi"("SJ Data String"=w95, "Mode"=T10."String to SJ Data Cluster") -> ("SJ Data Out"=w106:T2)  [unwired: 2 in, 1 out]
                n46 = global write "Synthetic_jet_global.vi" "SJ Data"(w106) -> ()
              }
            }
          }
          frame 2, Default {
            n47 = global read "Synthetic_jet_global.vi" "Channels to Analyse"() -> (w120:i32[])
            n48 = global read "Synthetic_jet_global.vi" "Num Bins"() -> (w121:i32)
          }
        }
        n49 = Equal?(x=w60, y=1) -> (x = y?=w58:bool)
        n50 = case shown="\"Post Process Raw Data File\"" w45 {
          tunnel: [w72 TRUE] -> w46
          tunnel: w44 -> [w70 _]
          frame "Take New Data" {
            n51 = Greater Than 0?(x=w70) -> (x > 0?=w72:bool)
            n52 = Not(x=w72) -> (.not. x?=w71:bool)
            n53 = global write "Meas_global.vi" "stop"(w71) -> ()
          }
          frame "Post Process Raw Data File" {
          }
        }
        n54 = Select(t="Selected Channels", s="Overide Channels?", f=w52) -> (s? t:f=w47:i32[])
        n55 = Select(t="Num Bins", s="Overide Bins?", f=w51) -> (s? t:f=w48:i32)
        n56 = Array Size(array=w47) -> (size(s)=w67:i32)
        n57 = case shown="1" w60 {
          tunnel: [w123 w127] -> w69
          tunnel: w68 -> [w123 _]
          tunnel: w67 -> [_ w125]
          tunnel: w48 -> [_ w124]
          frame 2, Default {
          }
          frame 1 {
            n58 = Initialize Array(T11 {"Start Time"=0.0, "End Time"=0.0, "Bin Number"=0, "Data Points"=0, "Shift"=[], "Stats"={"U"=0.0, "u^2"=0.0, "u^3"=0.0, "u^4"=0.0, "Skew_u"=0.0, "Kurt_u"=0.0, "% u'/U"=0.0}, "Channel Name"="", "Bin Centre"=0.0, "Symbol"=""} ("Bin Cluster"), w125, w124) -> (w127:T11[][])
          }
        }
        n59 = global write "Synthetic_jet_global.vi" "Num Bins"(w48) -> ()
        n60 = global write "Synthetic_jet_global.vi" "Channels to Analyse"(w47) -> ()
        n61 = Select(t="Create Bins", s=w58, f="Phase Average") -> (s? t:f=w62:string)
      }
      frame "Create Bins" {
        n62 = global read "Synthetic_jet_global.vi" "Num Bins"() -> (w134:i32)
        n63 = To Double Precision Float(number=w134) -> (double precision float=w143:dbl)
        n64 = Reciprocal(x=w128) -> (1/x=w133:ext)
        n65 = Divide(x=w133, y=w143) -> (x/y=w140:ext)
        "Bin Width" <- w140
        n66 = Subtract(x=w133, y=w140) -> (x-y=w141:ext)
        n67 = call-poly <vilib>:"Ramp Pattern.vi"("start"=w140, "end"=w133, "delta"=w140) -> ("Ramp Pattern"=w139:dbl[])  [unwired: 6 in, 2 out]
        n68 = call-poly <vilib>:"Ramp Pattern.vi"("start"=0.0, "end"=w141, "delta"=w140) -> ("Ramp Pattern"=w138:dbl[])  [unwired: 6 in, 2 out]
        n69 = for {
          tunnel: w139 -> [w159]
          tunnel: w138 -> [w158]
          tunnel: w137 -> [w157] mode=indexing
          tunnel: [w156] -> w136 mode=indexing
          tunnel: w135 -> [w149]
          tunnel: w130 -> [w148] mode=indexing
          tunnel: [w146] -> w129 mode=indexing
          i -> [w154]
          n70 = Index Array(array=w149, index=w148) -> (element=w147:T5)
          n71 = control-ref of="Engineering Values Scaled"() -> (w155:refnum<vi>)
          n72 = Unbundle By Name(w147) -> ("Inst name"=w146:string)
          n73 = for {
            tunnel: w157 -> [w169] mode=indexing
            tunnel: w159 -> [w164] mode=indexing
            tunnel: w158 -> [w163] mode=indexing
            tunnel: [w167] -> w156 mode=indexing
            tunnel: w147 -> [w160]
            i -> [w168]
            n74 = Build Array(w164, w163) -> (w165:dbl[])
            n75 = Unbundle By Name(w160) -> ("Inst name"=w162:string, "Symbol"=w161:string)
            n76 = call-poly <vilib>:"Mean.vi"("X"=w165) -> ("mean"=w166:dbl)  [unwired: 1 out]
            n77 = Bundle By Name(cluster=w169, "Bin Centre"=w166, "End Time"=w164, "Start Time"=w163, "Bin Number"=w168, "Channel Name"=w162, "Symbol"=w161) -> (w167:T11)
          }
          n78 = To Unsigned Long Integer(number=w154) -> (unsigned 32bit integer=w152:u32)
          n79 = control-ref of="Samples Per Bin"() -> (w151:refnum<vi>)
          n80 = property class="XYGraph (strict)"(reference=w155, "Active Plot"=w152, "Plot.Plot Name"=w146) -> (reference out=w153:refnum<vi>)  [unwired: 1 in, 1 out]
          n81 = property class="XYGraph (strict)"(reference=w151, "Active Plot"=w152, "Plot.Plot Name"=w146) -> (reference out=w150:refnum<vi>)  [unwired: 1 in, 1 out]
          n82 = Close Reference(reference=w153) -> ()  [unwired: 1 in, 1 out]
          n83 = Close Reference(reference=w150) -> ()  [unwired: 1 in, 1 out]
        }
        n84 = property on="Plot Channel" class="Ring (strict)"("Strings []"=w129) -> ()  [unwired: 2 in, 2 out]
      }
      frame "Phase Average" {
        n85 = local read "Bin Width"() -> (w180:dbl)
        n86 = Reciprocal(x=w170) -> (1/x=w181:ext)
        n87 = for {
          tunnel: w172 -> [w186]
          tunnel: w181 -> [w197]
          tunnel: w180 -> [w189]
          tunnel: w178 -> [w191] mode=indexing
          tunnel: w179 -> [w192]
          tunnel: [w190] -> w177 mode=indexing
          tunnel: [w188] -> w176 mode=indexing
          tunnel: w171 -> [w185] mode=indexing
          n88 = Index Array(array=w186, index=w185) -> (element=w184:T8)
          n89 = Unbundle By Name(w184) -> ("Time (s)"=w200:dbl[])
          n90 = Unbundle By Name(w184) -> ("Eng Values"=w187:dbl[], "Weighting"=w193:dbl[])
          n91 = Divide(x=w200, y=1.0) -> (x/y=w198:dbl[])
          n92 = Quotient & Remainder(x=w198, y=w197) -> (x-y*floor(x/y)=w196:ext[])  [unwired: 1 out]
          n93 = Quotient & Remainder(x=w196, y=w189) -> (floor(x/y)=w195:ext[])  [unwired: 1 out]
          n94 = To Long Integer(number=w195) -> (32bit integer=w194:i32[])
          n95 = for {
            tunnel: w194 -> [w223]
            tunnel: w187 -> [w209]
            tunnel: w193 -> [w207]
            tunnel: w192 -> [w222]
            tunnel: w191 -> [w211] mode=indexing
            tunnel: [w210] -> w190 mode=indexing
            tunnel: [w202] -> w188 mode=indexing
            i -> [w203]
            n96 = Unbundle By Name(w211) -> ("Data Points"=w205:i32, "Shift"=w220:dbl[])
            n97 = call "Search_1D_Array(I32).vi"("Array"=w223, "Element Data"=w203) -> ("Indicies of Elements"=w208:i32[])  [unwired: 6 in, 1 out]
            n98 = for {
              tunnel: w209 -> [w229]
              tunnel: w208 -> [w228] mode=indexing
              tunnel: [w227] -> w201 mode=indexing
              tunnel: w208 -> [w226] mode=indexing
              tunnel: w207 -> [w225]
              tunnel: [w224] -> w206 mode=indexing
              n99 = Index Array(array=w229, index=w228) -> (element=w227:dbl)
              n100 = Index Array(array=w225, index=w226) -> (element=w224:dbl)
            }
            n101 = call "Weighted_Fast_Response_Stats.vi"("U"=w201, "Weighting"=w206, "Use Weighting?"=TRUE, "Shift in"=w220, "Block No"=w222) -> ("U"=w212:dbl, "u^2"=w213:dbl, "u^3"=w214:dbl, "u^4"=w215:dbl, "Skew"=w216:dbl, "Kurt"=w217:dbl, "% u'/U"=w218:dbl, "Shift out"=w219:dbl[])  [unwired: 3 in]
            n102 = Array Size(array=w201) -> (size(s)=w204:i32)
            n103 = Add(x=w204, y=w205) -> (x+y=w202:i32)
            n104 = Bundle By Name(cluster=w211, "Data Points"=w202, "Stats.U"=w212, "Stats.u^2"=w213, "Stats.u^3"=w214, "Stats.u^4"=w215, "Stats.Skew_u"=w216, "Stats.Kurt_u"=w217, "Stats.% u'/U"=w218, "Shift"=w219) -> (w210:T11)
          }
        }
        n105 = Array Max & Min(array=w176) -> (min value=→"Min Num Data Points":i32)  [unwired: 3 out]
      }
      frame "Plot Graph" {
        n106 = for {
          tunnel: w255 -> [w292] mode=indexing
          tunnel: [w286] -> w254 mode=indexing
          tunnel: [w280] -> w239 mode=indexing
          tunnel: [w285] -> w247 mode=indexing
          tunnel: [w284] -> w246 mode=indexing
          tunnel: "Plot Data" -> [w283]
          tunnel: [w282] -> w241 mode=indexing
          tunnel: [w281] -> w238 mode=concatenating
          tunnel: [w280] -> w240 mode=concatenating
          tunnel: [w279] -> _ mode=concatenating
          tunnel: [w278] -> w235
          n107 = for {
            tunnel: [w298] -> w288 mode=indexing
            tunnel: [w297] -> w280 mode=indexing
            tunnel: w292 -> [w295] mode=indexing
            tunnel: [w296] -> w285 mode=indexing
            tunnel: w283 -> [w294]
            tunnel: [w293] -> w279 mode=indexing
            n108 = case shown="\"U\", Default" w294 {
              tunnel: w295 -> [w300 w302 w304 w306 w308 w310 w312]
              tunnel: [w299 w301 w303 w305 w307 w309 w311] -> w293
              frame "U", Default {
                n109 = Unbundle By Name(w300) -> ("Stats.U"=w299:dbl)
              }
              frame "u^2" {
                n110 = Unbundle By Name(w302) -> ("Stats.u^2"=w301:dbl)
              }
              frame "u^3" {
                n111 = Unbundle By Name(w304) -> ("Stats.u^3"=w303:dbl)
              }
              frame "u^4" {
                n112 = Unbundle By Name(w306) -> ("Stats.u^4"=w305:dbl)
              }
              frame "Skew_u" {
                n113 = Unbundle By Name(w308) -> ("Stats.Skew_u"=w307:dbl)
              }
              frame "Kurt_u" {
                n114 = Unbundle By Name(w310) -> ("Stats.Kurt_u"=w309:dbl)
              }
              frame "% u'/U" {
                n115 = Unbundle By Name(w312) -> ("Stats.% u'/U"=w311:dbl)
              }
            }
            n116 = Unbundle By Name(w295) -> ("Bin Number"=w298:i32, "Stats.U"=w297:dbl, "Data Points"=w296:i32)
          }
          n117 = global read "Synthetic_jet_global.vi" "Num Bins"() -> (w289:i32)
          n118 = To Double Precision Float(number=w289) -> (double precision float=w278:dbl)
          n119 = To Double Precision Float(number=w288) -> (double precision float=w287:dbl[])
          n120 = Compound Arithmetic op=MULTIPLY(invert w278, w287, 360.0 ("value")) -> (w281:dbl[])
          n121 = call-poly <vilib>:"Scale.vi"("X"=w280) -> ("Y=(X-offset)/scale"=w291:dbl[])  [unwired: 3 out]
          n122 = Bundle(w281, "Y=(X-offset)/scale"=w291) -> (w286:cluster{dbl[], "Y=(X-offset)/scale":dbl[]})  [unwired: 1 in]
          n123 = Bundle(w281, w285) -> (w284:cluster{dbl[], i32[]})  [unwired: 1 in]
          n124 = Bundle(w281, w279) -> (w282:cluster{dbl[], dbl[]})  [unwired: 1 in]
        }
        "Engineering Values Scaled" <- w254
        "U" <- w239
        "Data Points" <- w247
        "Samples Per Bin" <- w246
        n125 = local read "Min Num Data Points"() -> (w250:i32)
        n126 = Greater?(x=w250, y=500) -> (0:w249:bool)
        n127 = global write "Meas_global.vi" "stop"(w249) -> ()
        n128 = Decrement(x=w235) -> (x-1=w231:dbl)
        n129 = Index Array(array=w241, index="Plot Channel") -> (element=→"Engineering Values":cluster{dbl[], dbl[]})
        n130 = Build Array(w240, w238) -> (w237:dbl[][])
        n131 = global read "Meas_global.vi" "Processing last block?"() -> (w248:bool)
        n132 = Transpose 2D Array(2D array=w237) -> (transposed array=w236:dbl[][])
        n133 = Delete From Array(array=w236, length=w231, index (row)=0) -> (deleted portion=w232:dbl[][], array with subset deleted=w234:dbl[][])  [unwired: 1 in]
        n134 = case shown="True" "Write out PA data?" {
          tunnel: w241 -> [_ _]
          tunnel: w234 -> [_ w267]
          tunnel: w232 -> [_ w266]
          tunnel: w230 -> [_ w265]
          frame False {
          }
          frame True {
            w257 = "_FILE_" ("string")
            (unwired) ".xls" ("string")
            n135 = Path To String(path=w265) -> (string=w263:string)
            n136 = Match Pattern(string=w263, regular expression="Raw_Measurements\\" ("string")) -> (after substring=w261:string)  [unwired: 1 in, 3 out]
            n137 = Match Pattern(string=w261, regular expression="_xls\\" ("string")) -> (after substring=w258:string)  [unwired: 1 in, 3 out]
            n138 = Concatenate Strings("U" ("string"), w257, w258) -> (w270:string)
            n139 = Build Path(base path=path "C:/Users/Nick Martin/Desktop/mike_jets_data", name or relative path=w270) -> (appended path=w271:path)
            n140 = call-poly <vilib>:"Write To Spreadsheet File.vi"("format (%.3f)"="%.8f", "append to file? (new file:F)"=FALSE, "2D data"=w266, "file path (dialog if empty)"=w271) -> ()  [unwired: 4 in, 1 out]
            n141 = Concatenate Strings("Vin" ("string"), w257, w258) -> (w274:string)
            n142 = Build Path(base path=path "C:/Users/Nick Martin/Desktop/mike_jets_data", name or relative path=w274) -> (appended path=w275:path)
            n143 = call-poly <vilib>:"Write To Spreadsheet File.vi"("format (%.3f)"="%.8f", "append to file? (new file:F)"=FALSE, "2D data"=w267, "file path (dialog if empty)"=w275) -> ()  [unwired: 4 in, 1 out]
          }
        }
      }
      frame "Save Data" {
        n144 = local read "Data Points"() -> (w315:i32[][])
        n145 = local read "U"() -> (w320:dbl[][])
        n146 = for {
          tunnel: w320 -> [w337] mode=indexing
          shift-right: [w357] -> w318
          shift-left: w319 -> [w358]
          shift-right: [w356] -> w316
          shift-left: w317 -> [w335]
          tunnel: w315 -> [w351] mode=indexing
          tunnel: w314 -> [w334] mode=indexing
          tunnel: w313 -> [w333]
          w354 = i16 8 ("precision (6)")
          n147 = Index Array(array=w333, index=w334) -> (element=w332:T5)
          n148 = Array Max & Min(array=w351) -> (max value=w349:i32, min value=w347:i32)  [unwired: 2 out]
          n149 = Array Max & Min(array=w337) -> (max value=w331:dbl, min value=w325:dbl)  [unwired: 2 out]
          n150 = call-poly <vilib>:"Mean.vi"("X"=w337) -> ("mean"=w353:dbl)  [unwired: 1 out]
          n151 = Unbundle By Name(w332) -> ("Symbol"=w329:string, "Inst Array"=w341:T7)
          n152 = Number To Decimal String(number=w349) -> (decimal integer string=w348:string)  [unwired: 1 in]
          n153 = Number To Decimal String(number=w347) -> (decimal integer string=w345:string)  [unwired: 1 in]
          n154 = Number To Fractional String(number=w353, precision (6)=w354) -> (F-format string=w352:string)  [unwired: 2 in]
          n155 = Number To Fractional String(number=w331, precision (6)=w354) -> (F-format string=w326:string)  [unwired: 2 in]
          n156 = Number To Fractional String(number=w325) -> (F-format string=w324:string)  [unwired: 3 in]
          n157 = Concatenate Strings("Synthetic_Jet:PA_Mean_U:", w329) -> (w344:string)
          n158 = Concatenate Strings("Synthetic_Jet:PA_Max_U:", w329) -> (w328:string)
          n159 = Concatenate Strings("Synthetic_Jet:PA_Min_U:", w329) -> (w327:string)
          n160 = Concatenate Strings("Synthetic_Jet:PA_Data_Points_Max:", w329) -> (w343:string)
          n161 = Concatenate Strings("Synthetic_Jet:PA_Data_Points_Min:", w329) -> (w342:string)
          n162 = Build Array(w328, w327, w344, w343, w342) -> (w338:string[])
          n163 = Build Array(w326, w324, w352, w348, w345) -> (w340:string[])
          n164 = case shown="\"LDA\"" w341 {
            tunnel: [w371 w377] -> w336
            tunnel: w340 -> [w370 w377]
            tunnel: [w372 w376] -> w339
            tunnel: w338 -> [w374 w376]
            tunnel: w329 -> [w360 _]
            tunnel: w337 -> [w369 _]
            frame "LDA" {
              w366 = i16 8 ("precision (6)")
              n165 = local read "Bin Width"() -> (w368:dbl)
              n166 = call "Get_Characteristic_Velocity.vi"("dt (bin width)"=w368, "Velocity"=w369) -> ("Uo"=w367:dbl, "Tb/T"=w365:dbl)  [unwired: 6 in, 2 out]
              n167 = Number To Fractional String(number=w367, precision (6)=w366) -> (F-format string=w364:string)  [unwired: 2 in]
              n168 = Number To Fractional String(number=w365, precision (6)=w366) -> (F-format string=w363:string)  [unwired: 2 in]
              n169 = Concatenate Strings("Synthetic_Jet:PA_Uo:", w360) -> (w373:string)
              n170 = Concatenate Strings("Synthetic_Jet:PA_Tb/T:", w360) -> (w361:string)
              n171 = Build Array (concatenate)(w370, w364, w363) -> (w371:string[])
              n172 = Build Array (concatenate)(w374, w373, w361) -> (w372:string[])
            }
            frame "Analogue", Default {
            }
          }
          n173 = Build Array (concatenate)(w358, w339) -> (w357:string[])
          n174 = Build Array (concatenate)(w335, w336) -> (w356:string[])
        }
      }
      frame "Cross Correlation" {
        n175 = local read "U"() -> (w378:dbl[][])
        n176 = call "Chs_to_Correlate.vi"("Valid Ch to correlate"=w386) -> ("Correlation Pairs"=w385:i32[][])
        n177 = for {
          tunnel: w378 -> [w429]
          tunnel: w385 -> [w430] mode=indexing
          tunnel: w384 -> [w428]
          shift-right: [w399] -> w382
          shift-left: w383 -> [w398]
          shift-right: [w389] -> w380
          shift-left: w379 -> [w388]
          w394 = i16 8 ("precision (6)")
          w427 = 0 ("disabled index (col)")
          n178 = Index Array(array=w430) -> (element #1=w417:i32, element #2=w416:i32)  [unwired: 2 in]
          n179 = Index Array(array=w428, index (row)=w417, index (col)=w427) -> (element=w426:T11)
          n180 = Index Array(array=w428, index (row)=w416, index (col)=w427) -> (element=w425:T11)
          n181 = Index Array(array=w429, index (row)=w417) -> (element=w412:dbl[])  [unwired: 1 in]
          n182 = Index Array(array=w429, index (row)=w416) -> (element=w410:dbl[])  [unwired: 1 in]
          n183 = Unbundle By Name(w426) -> ("Symbol"=w424:string)
          n184 = Unbundle By Name(w425) -> ("Symbol"=w423:string)
          n185 = call "Normalise_Signal.vi"("x"=w412) -> ("(x-X)/sigma"=w411:dbl[])  [unwired: 4 in]
          n186 = call "Normalise_Signal.vi"("x"=w410) -> ("(x-X)/sigma"=w409:dbl[])  [unwired: 4 in]
          n187 = global read "Synthetic_jet_global.vi" "Num Bins"() -> (w407:i32)
          n188 = Concatenate Strings(w424, "_cross_" ("string"), w423) -> (w402:string)
          n189 = call-poly <vilib>:"CrossCorrelation.vi"("normalization"=enum32{"none", "unbiased", "biased"}."biased", "algorithm"=enum32{"direct", "frequency domain"}."frequency domain", "Y"=w409, "X"=w411) -> ("Rxy"=w413:dbl[])  [unwired: 6 in, 1 out]
          n190 = Index Array(array=w413, index=w407) -> (element=w397:dbl)
          n191 = call <vilib>:"Peak Detector.vi"("width"=3, "X"=w413) -> ("Amplitudes"=w418:dbl[], "Locations"=w420:dbl[])  [unwired: 5 in, 3 out]
          n192 = Array Max & Min(array=w418) -> (max value=w396:dbl, max index (indices)=w419:i32)  [unwired: 2 out]
          n193 = for {
            tunnel: w402 -> [w432]
            tunnel: string[] ["Synthetic_Jet:PA_Corr_Coeff:", "Synthetic_Jet:PA_Corr_Coeff_Max:", "Synthetic_Jet:Phase_Lag:"] ("Corr Channels") -> [w433] mode=indexing
            tunnel: [w431] -> w400 mode=indexing
            n194 = Concatenate Strings(w433, w432) -> (w431:string)
          }
          n195 = Index Array(array=w420, index=w419) -> (element=w403:dbl)
          n196 = To Double Precision Float(number=w407) -> (double precision float=w404:dbl)
          n197 = Subtract(x=w403, y=w404) -> (x-y=w408:dbl)
          n198 = Divide(x=w408, y=w404) -> (x/y=w406:dbl)
          n199 = Multiply(x=w406, y=360.0) -> (x*y=w395:dbl)
          n200 = Number To Fractional String(number=w397, precision (6)=w394) -> (F-format string=w393:string)  [unwired: 2 in]
          n201 = Number To Fractional String(number=w396, precision (6)=w394) -> (F-format string=w392:string)  [unwired: 2 in]
          n202 = Number To Fractional String(number=w395, precision (6)=w394) -> (F-format string=w391:string)  [unwired: 2 in]
          n203 = Build Array(w393, w392, w391) -> (w390:string[])
          n204 = Build Array (concatenate)(w398, w400) -> (w399:string[])
          n205 = Build Array (concatenate)(w388, w390) -> (w389:string[])
        }
      }
      frame "Fourier Decomposition" {
        n206 = local read "Bin Width"() -> (w435:dbl)
        n207 = local read "U"() -> (w450:dbl[][])
        n208 = for {
          tunnel: w450 -> [w479] mode=indexing
          shift-right: [w499] -> w448
          shift-left: w449 -> [w500]
          shift-right: [w458] -> w439
          shift-left: w438 -> [w457]
          tunnel: w434 -> [w482]
          tunnel: w435 -> [w477]
          tunnel: [w496] -> w446 mode=indexing
          tunnel: [w488] -> w444 mode=indexing
          tunnel: [w484] -> w442 mode=indexing
          tunnel: w437 -> [w456]
          tunnel: w436 -> [w455] mode=indexing
          w464 = i16 10 ("precision (6)")
          w478 = 3 ("length")
          w485 = 0 ("index")
          n209 = Index Array(array=w456, index=w455) -> (element=w454:T5)
          n210 = Array Size(array=w479) -> (size(s)=w487:i32)
          n211 = Reciprocal(x=w482) -> (1/x=w486:ext)
          n212 = call-poly <vilib>:"Scale.vi"("X"=w479) -> ("Y=(X-offset)/scale"=w476:dbl[], "scale"=w469:dbl, "offset"=w468:dbl)  [unwired: 1 out]
          n213 = Unbundle By Name(w454) -> ("Symbol"=w491:string)
          n214 = call-poly <vilib>:"Ramp Pattern.vi"("exclude end?"=TRUE, "end"=w486, "samples"=w487) -> ("Ramp Pattern"=w475:dbl[])  [unwired: 7 in, 1 out]
          n215 = call <vilib>:"Amplitude and Phase Spectrum.vi"("dt"=w477, "unwrap phase (T)"=TRUE, "Signal (V)"=w476) -> ("df"=w474:dbl, "Amp Spectrum Phase (radians)"=w472:dbl[], "Amp Spectrum Mag (Vrms)"=w471:dbl[])
          "phiK" <- w472
          "Ak" <- w471
          n216 = Build Array(w469, w468) -> (w467:dbl[])
          n217 = Array Size(array=w471) -> (size(s)=w498:i32)
          n218 = Number To Fractional String(number=w467, precision (6)=i16 10) -> (F-format string=w461:string[])  [unwired: 2 in]
          n219 = Multiply(x=w498, y=w474) -> (x*y=w497:dbl)
          n220 = call-poly <vilib>:"Ramp Pattern.vi"("exclude end?"=TRUE, "end"=w497, "samples"=w498) -> ("Ramp Pattern"=w480:dbl[])  [unwired: 7 in, 1 out]
          "fk" <- w480
          n221 = Concatenate Strings("Synthetic_Jet:Fourier_Coeff_Scale:", w491) -> (w489:string)
          n222 = Concatenate Strings("Synthetic_Jet:Fourier_Coeff_Offset:", w491) -> (w490:string)
          n223 = Concatenate Strings("Synthetic_Jet:Fourier_Coeff_Amp_1:", w491) -> (w506:string)
          n224 = Concatenate Strings("Synthetic_Jet:Fourier_Coeff_Phase_1:", w491) -> (w505:string)
          n225 = Concatenate Strings("Synthetic_Jet:Fourier_Coeff_Amp_2:", w491) -> (w504:string)
          n226 = Concatenate Strings("Synthetic_Jet:Fourier_Coeff_Phase_2:", w491) -> (w503:string)
          n227 = Concatenate Strings("Synthetic_Jet:Fourier_Coeff_Amp_3:", w491) -> (w502:string)
          n228 = Concatenate Strings("Synthetic_Jet:Fourier_Coeff_Phase_3:", w491) -> (w501:string)
          n229 = Bundle("Ramp Pattern"=w480, "Amp Spectrum Mag (Vrms)"=w471) -> (w496:T4)  [unwired: 1 in]
          n230 = Bundle("Ramp Pattern"=w480, "Amp Spectrum Phase (radians)"=w472) -> (w488:T12)  [unwired: 1 in]
          n231 = Multiply(x=6.283185307179586, y=w480) -> ()  [unwired: 1 out]
          n232 = Build Array(w489, w490, w506, w505, w504, w503, w502, w501) -> (w495:string[])
          n233 = Array Subset(array=w472, index=w485, length=w478) -> (w470:dbl[])
          n234 = Array Subset(array=w471, index=w485, length=w478) -> (w465:dbl[])
          n235 = Number To Fractional String(number=w470, precision (6)=w464) -> (F-format string=w462:string[])  [unwired: 2 in]
          n236 = Number To Fractional String(number=w465, precision (6)=w464) -> (F-format string=w463:string[])  [unwired: 2 in]
          n237 = Interleave 1D Arrays(w463, w462) -> (w460:string[])
          n238 = call "Inverse_Auto_Amp_Spectra.vi"("df"=w474, "t"=w475, "Amp Spectrum Mag (Vrms)"=w465, "Amp Spectrum Phase (radians)"=w470) -> ("X"=w473:dbl[])  [unwired: 6 in, 1 out]
          n239 = Build Array (concatenate)(w461, w460) -> (w459:string[])
          n240 = Build Array (concatenate)(w500, w495) -> (w499:string[])
          n241 = Build Array (concatenate)(w457, w459) -> (w458:string[])
          n242 = Bundle("Ramp Pattern"=w475, "X"=w473) -> (w484:cluster{"Ramp Pattern":dbl[], "X":dbl[]})  [unwired: 1 in]
        }
        n243 = Index Array(array=w442, index="index") -> (element=→"XY Graph":cluster{"Ramp Pattern":dbl[], "X":dbl[]})
        n244 = Index Array(array=w444, index="index") -> (element=→"Phase":T12)
        n245 = Index Array(array=w446, index="index") -> (element=→"Amp":T4)
      }
    }
  }
  "Plug in values" <- w3
  "Plug in titles" <- w4
